vi "main_004.vi"() -> ()   [LabVIEW 2017]
uses:
  ISEGNHQxxu/iseg NHQ VISA Control.ctl
  <vilib>/Analysis/1siggen.llb/Ramp Pattern by Samples.vi
  <vilib>/Utility/file.llb/Read From Spreadsheet File (DBL).vi
  <vilib>/Utility/file.llb/Write Delimited Spreadsheet (string).vi
  <vilib>/Utility/file.llb/Write Delimited Spreadsheet (DBL).vi
  <vilib>/Platform/browser.llb/Open URL in Default Browser (path).vi
  <vilib>/Analysis/NI_AALBase.lvlib
  Newport ESP301/Newport ESP301.lvlib
panel:
  in  "continous acq.":bool
  in  "snap":bool
  in  "dark":bool
  in  "savebin":bool
  in  "savepng":bool
  in  "count?":bool
  in  "dark?":bool
  in  "threshold":i32=100
  in  "t_exp":dbl=0.10000637173652649 caption="Exposure time [s]"
  in  "dark_load":bool
  in  "frames":i32=300
  in  "avg[t] acc[f]":bool
  in  "Value in":dbl=2.0 caption="binning"
  in  "stop":bool
  out "Slide":dbl(slide)=0.9966666666666667 scale=0.0..1.0
  in  "open base path":bool
  in  "Path":path=path "W:/fsPPM/data/2019/11/191112"
  in  "Tab Control":T1(tab)=enum."delayscan"
  out "Waveform Chart":dbl(graph)=8402498.700000005
  in  "array size":i32=50
  out "noise-o-meter":dbl=7.252741087138157 format="%.1g"
  out "Actual Voltage":dbl[unit]=-90.03 format="%.2f"
  in  "volt_set":bool
  in  "Nominal Voltage":sgl=90.0 min=0 max=1000 step=1 format="%.2f"
  out "delayscan_time/step":dbl format="%.2f"
  out "delayscan_steps":i32
  in  "esp_rel_delta_fs":dbl=0.015 caption="delta [fs]" min=0.0
  in  "delayscan_go":bool
  in  "waypoints":string[][](table)=[["-500", "50"], ["500", ""], ["", ""]]
  in  "delayscan_header":string="DelayScan01" caption="header"
  in  "iterations":i32=1
  out "XY Graph":cluster{"Array":dbl[], dbl[]}(graph)={"Array"=[-500.0, -450.0, -400.0, -350.0, -300.0, -250.0, -200.0, -150.0, -100.0, -50.0, 0.0, 50.0, 100.0, 150.0, 200.0, 250.0, 300.0, 350.0, 400.0, 450.0, 500.0], [74.7680418855, 74.77553669695, 0.0, 0.0, 0.0, 0.0, 0.0, 0.0, 0.0, 0.0, 0.0, 0.0, 0.0, 0.0, 0.0, 0.0, 0.0, 0.0, 0.0, 0.0, 0.0]}
  in  "delayscan_stop":bool
  in  "esp_abs_dest":dbl=74.87296924580001 caption="[mm]"
  out "t0 @":dbl=74.84299 format="%.6g"
  in  "esp_set_t0":bool
  in  "esp_abs_time":dbl=200.0 caption="[fs]"
  in  "esp_rel_delta":dbl=0.015 caption="delta [mm]" min=0.0
  in  "esp_abs_go":bool
  in  "esp_rel-":bool
  in  "esp_rel+":bool
  out "delay_pos":dbl=74.77555 caption="[mm]" format="%.6g"
  out "esp_pos_fs":dbl=-449.91125160329966 caption="[fs]" format="%.6g"
  in  "delayscan_pause":bool caption="pause"
  out "duration":dbl format="%<%H:%M:%S>t"
  out "Slide 2":dbl(slide)=0.999 scale=0.0..1.0
  in  "meas_stop_volt":bool
  in  "meas_start_volt":bool
  in  "head":string="PowerVoltScan1"
  in  "volt_start":dbl format="%0.2f"
  in  "volt_end":dbl=1.0 format="%0.2f"
  in  "volt_samples":i32=128
  in  "iterations 2":i32
  in  "move2com":bool
  in  "meas_start_XY":bool
  in  "showcom":bool
  in  "VISA ISEG":refnum<visa-resource-name>="COM3"
  in  "Channel (A)":enum16{"A", "B"}(ring)=enum."B"
  out "error out":errorcluster
  in  "volt_timeout":u32=6000
  in  "volt_threshold":sgl=2.0 max=4000 format="%.2f"
  in  "esp_axis":i32=1 caption="ESP Axis" min=1 max=3
  in  "esp_visa":refnum<visa-resource-name>="COM2" caption="ESP VISA"
  out "esp301":errorcluster
  in  "Serial Link (RS232)":enum16{"RS232", "USB"}(ring)
  out "captured":dbl[][](graph)
  out "live":dbl[][](graph)
  in  "close":bool
  # "camera"
  # "voltage supply"
  # "Move absolute"
  # "Move relative"
  # "Axis1"
  # "Axis2"
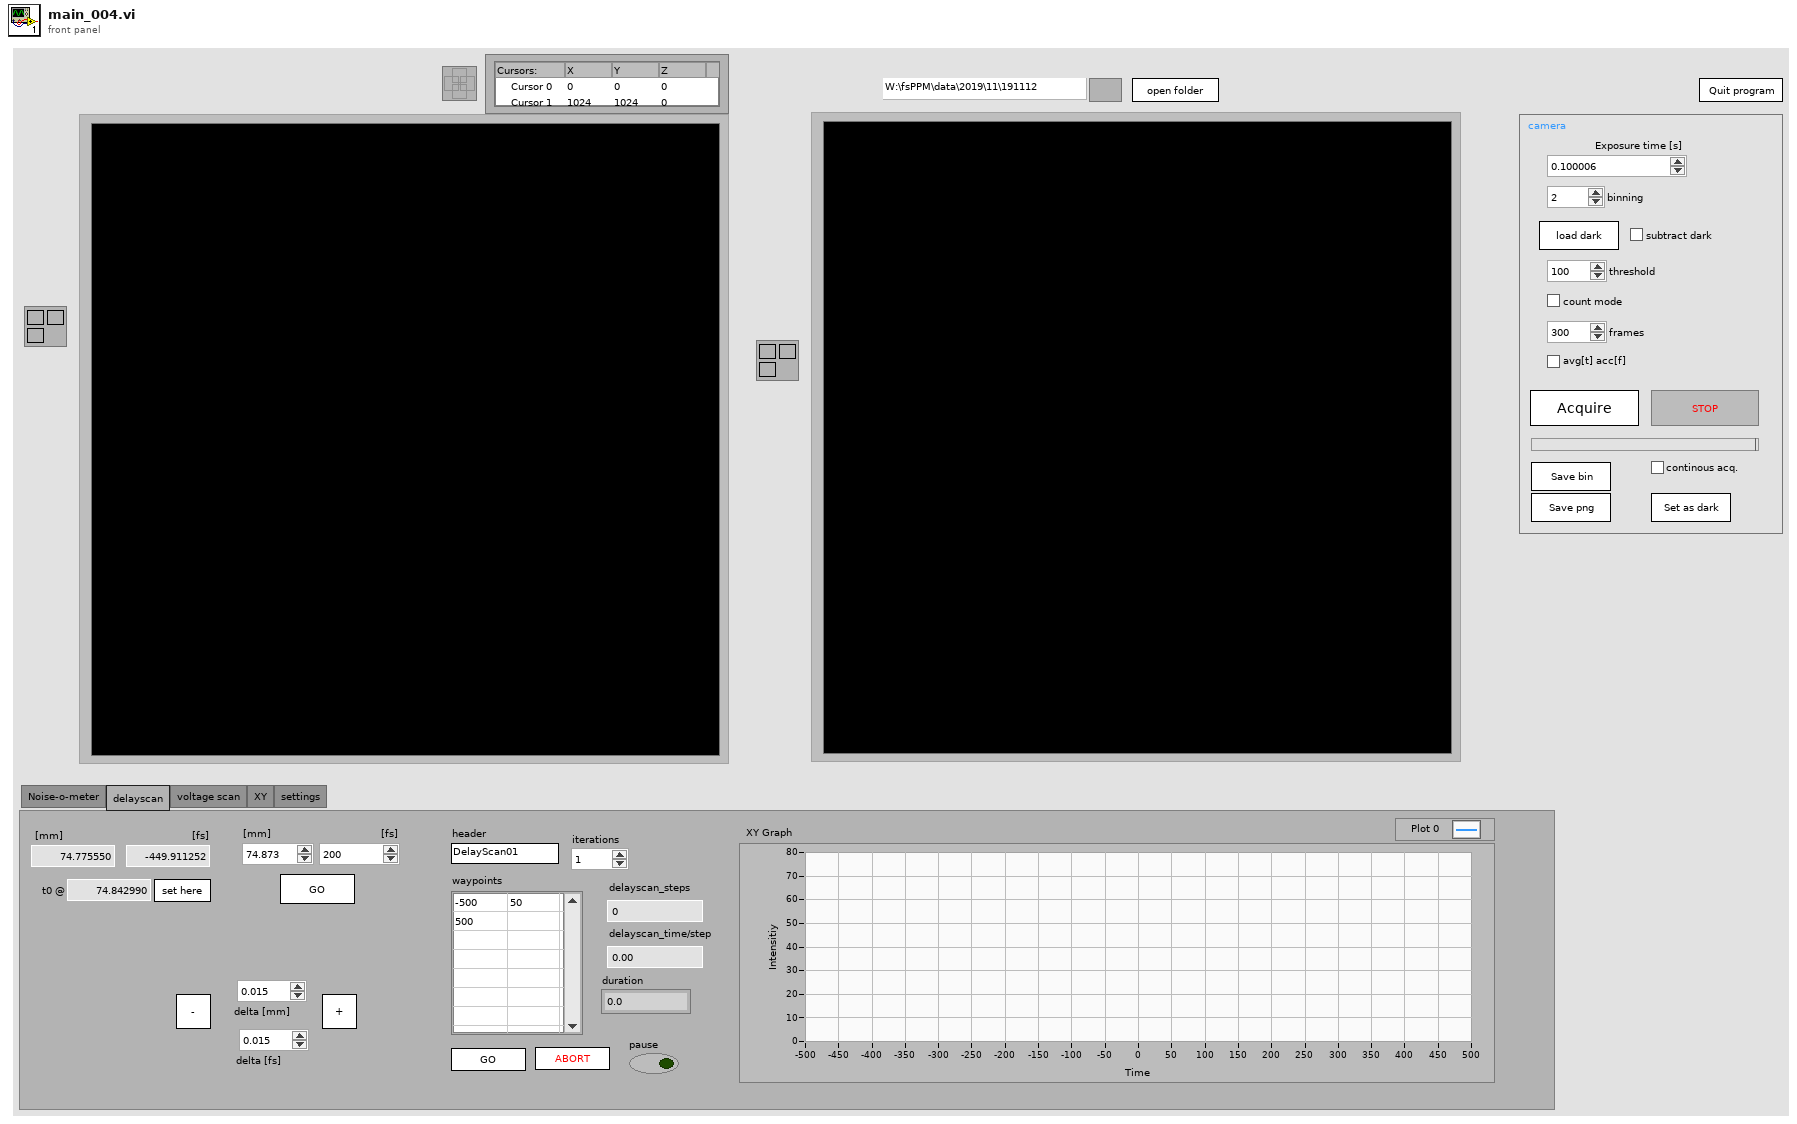
[diagram p1: front panel]
types:
  T1 = enum32{"Noise-o-meter", "delayscan", "voltage scan", "XY", "settings"}
  T2 = typedef "Image Type" = u32
  T3 = typedef "IMAQ Image.ctl" = refnum<image>
  T4 = cluster{"height":u32, "width":u32, "datatype":u32}
  T5 = cluster{"Axis1 moving":bool, "Axis2 moving":bool, "Axis3 moving":bool, "Axis4 moving":bool, "Motor Power of at least one axis":bool, "Reserved":bool, "Reserved":bool, "Reserved":bool, "Axis5 moving 2":bool, "Axis6 moving 2":bool, "Reserved":bool, "Reserved":bool, "Motor Power of at least one axis":bool, "Reserved":bool, "Reserved":bool, "Reserved":bool}
  T6 = typedef "iseg NHQ VISA Control.ctl" = cluster{"VISA Resource Name":refnum<visa-resource-name>, "FP Notation":bool, "Maximum Voltage":u32, "Maximum Current":u32}
  T7 = typedef "LVCursorListTypeDef.ctl" = cluster{"Name":string, "Color":u32, "Style":u8, "Point Style":u8, "Name Visible":bool, "Allow Drag":bool, "Cursor Mode":u32, "Plot":i32, "Index":i32, "Position":cluster{"X":dbl, "Y":dbl}, "X Scale":u32, "Y Scale":u32, "Watch Plots":i32[], "Watch All Plots":bool, "Plot Area":i32, "Label Offset":cluster{"X":dbl, "Y":dbl}}[]
  T8 = cluster{"Name":string, "Color":u32, "Style":u8, "Point Style":u8, "Name Visible":bool, "Allow Drag":bool, "Cursor Mode":u32, "Plot":i32, "Index":i32, "Position":cluster{"X":dbl, "Y":dbl}, "X Scale":u32, "Y Scale":u32, "Watch Plots":i32[], "Watch All Plots":bool, "Plot Area":i32, "Label Offset":cluster{"X":dbl, "Y":dbl}}
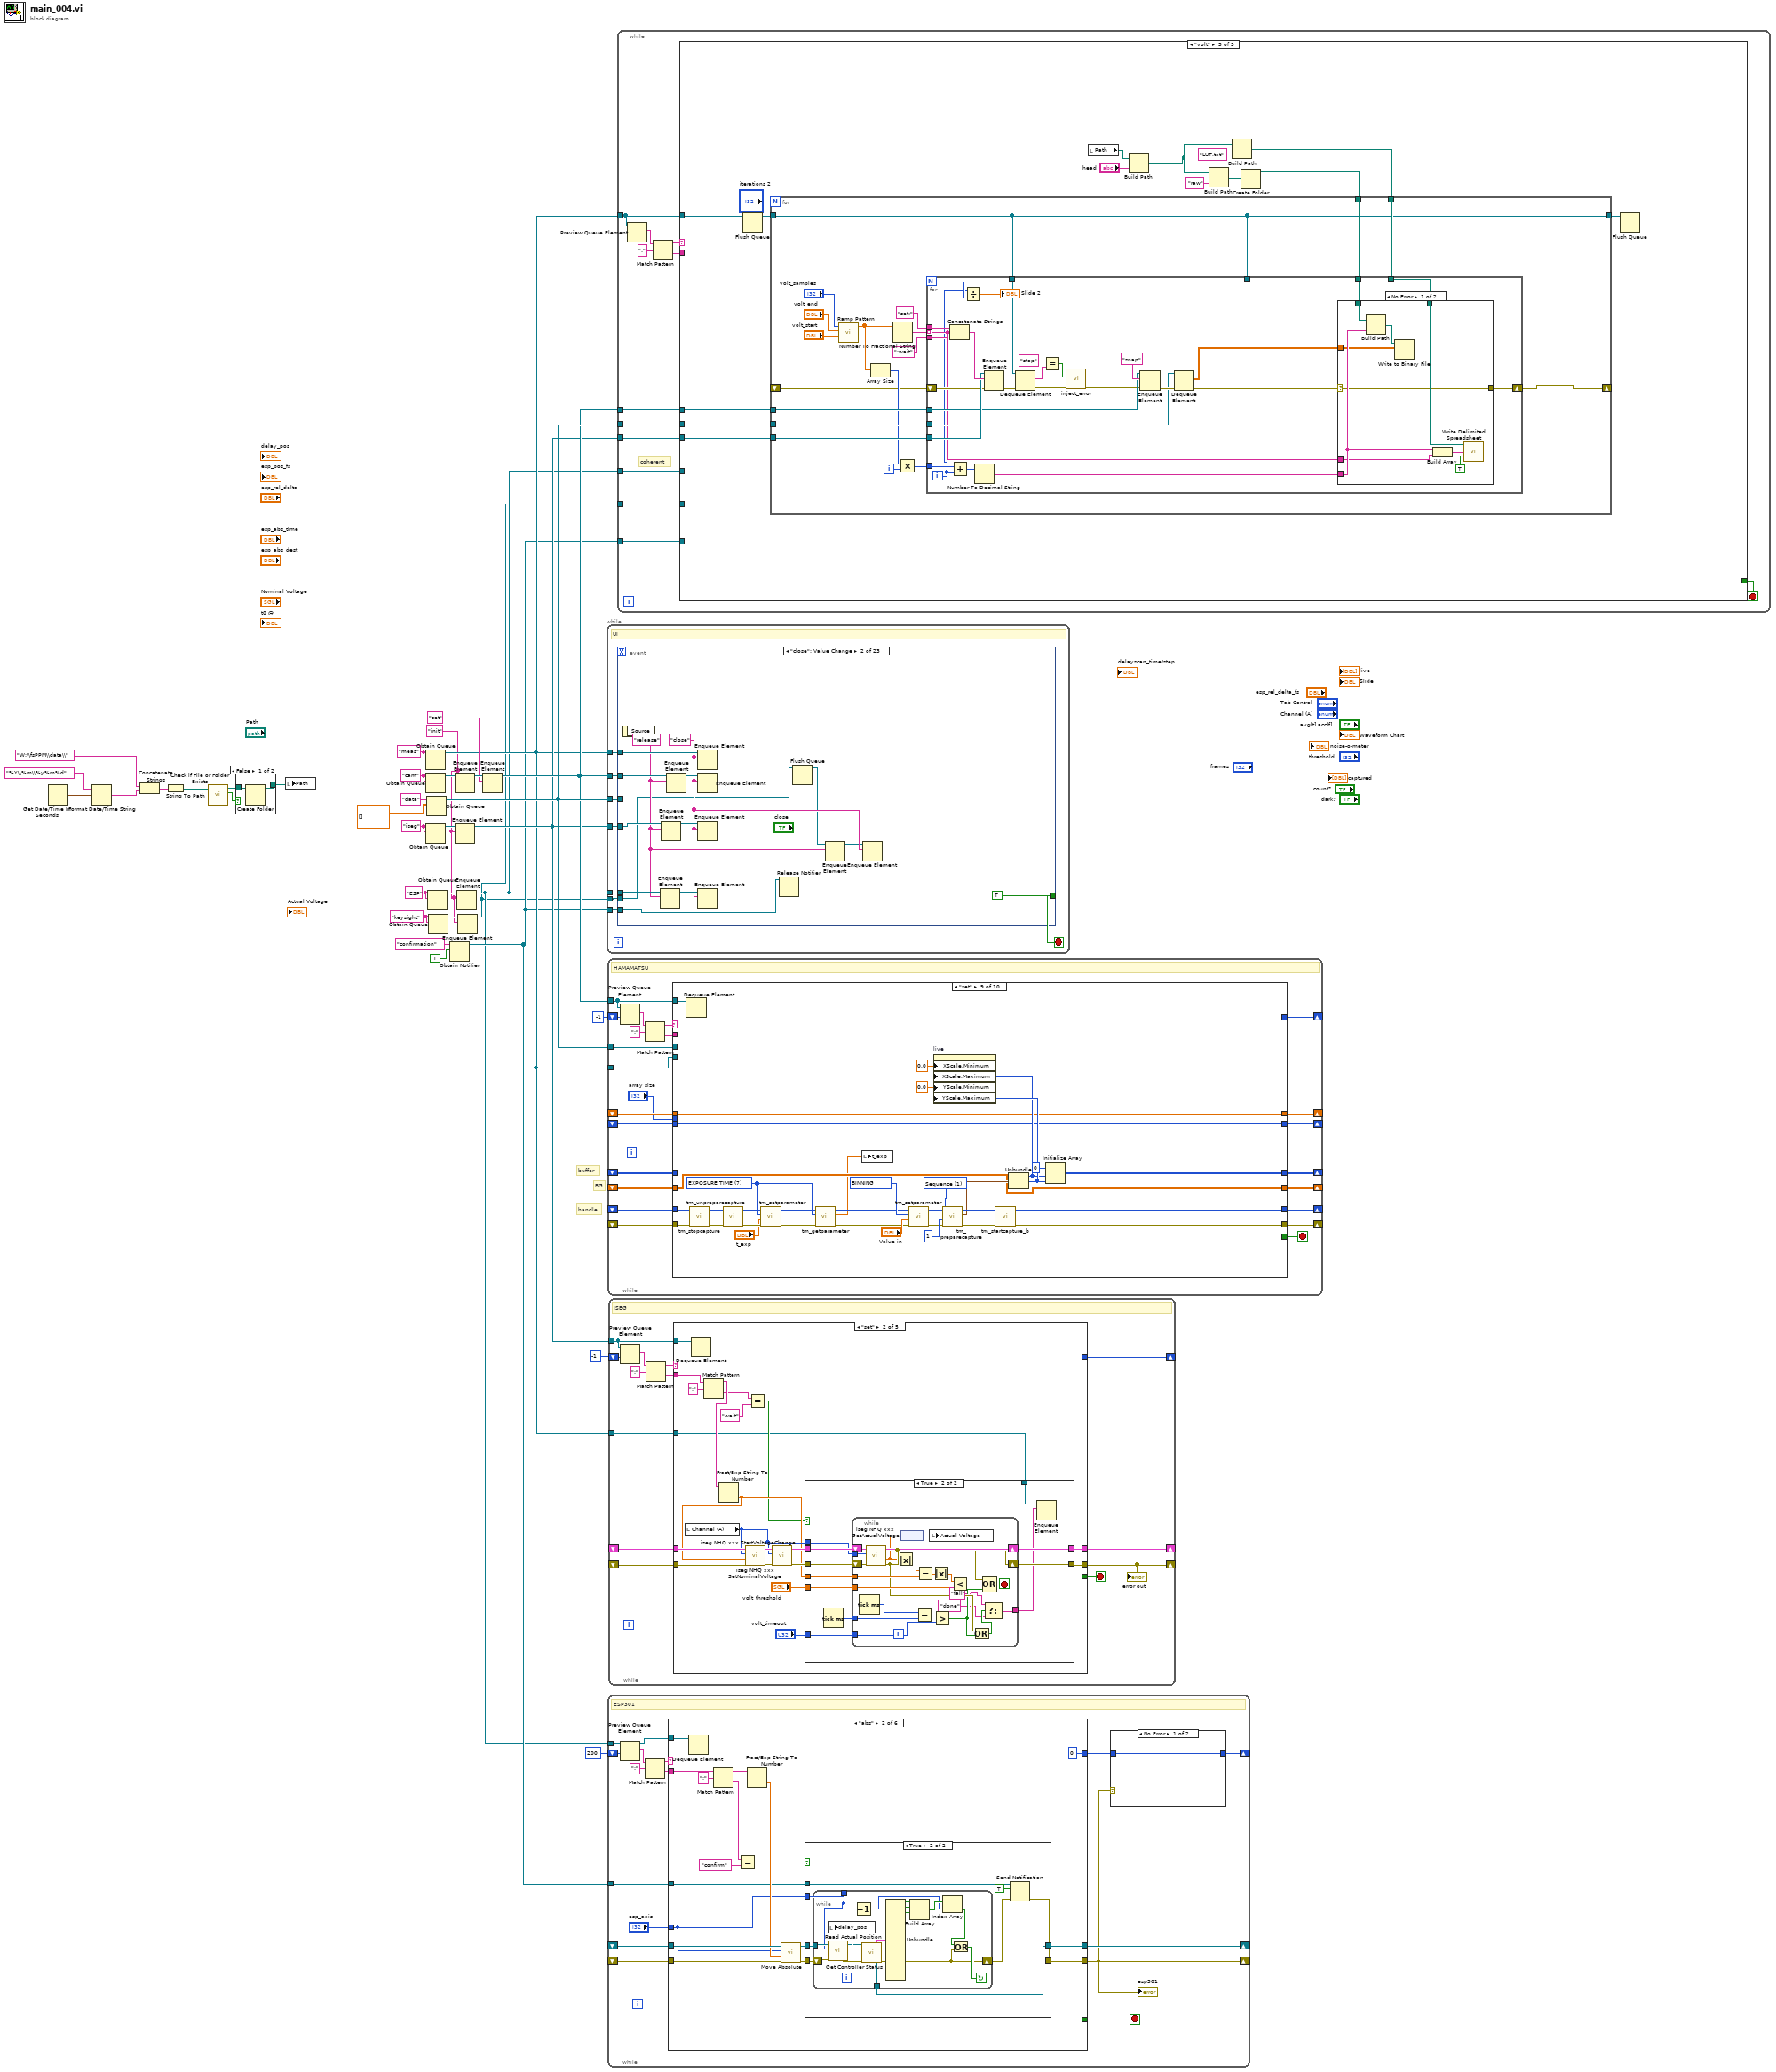
[diagram p0: block diagram]
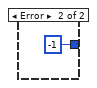
[diagram p3: hidden frame]
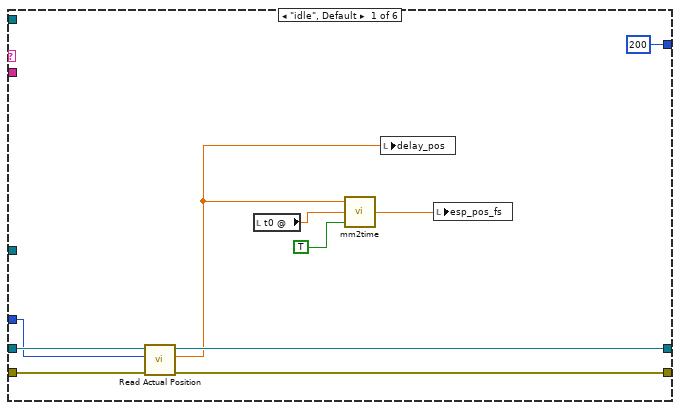
[diagram p4: hidden frame]
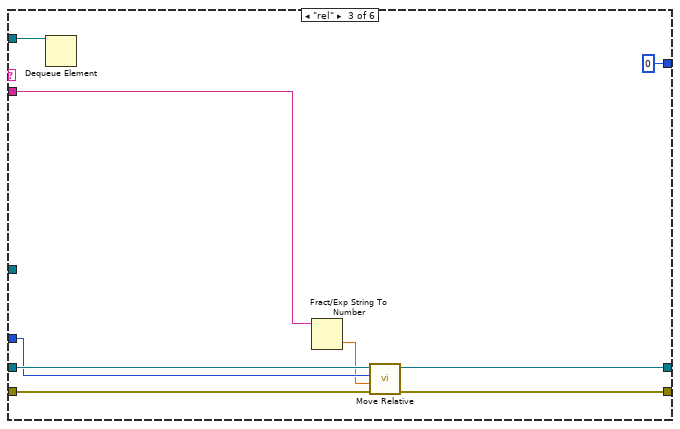
[diagram p6: hidden frame]
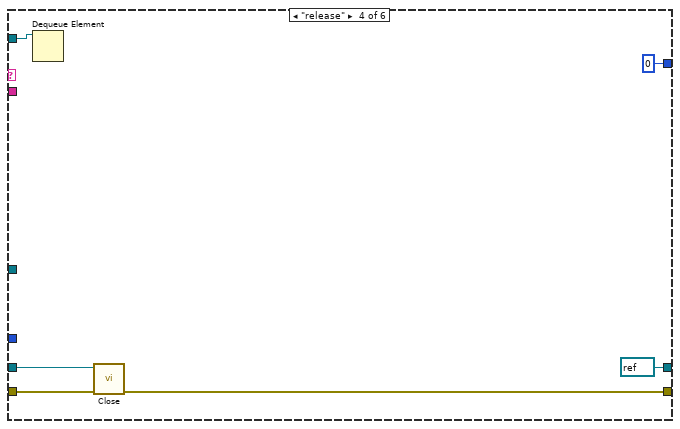
[diagram p7: hidden frame]
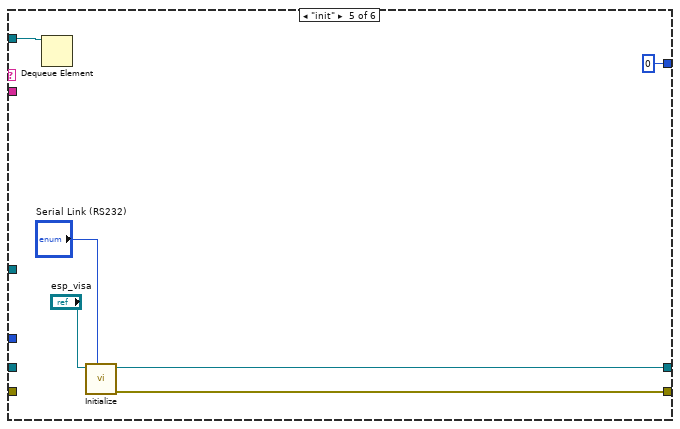
[diagram p8: hidden frame]
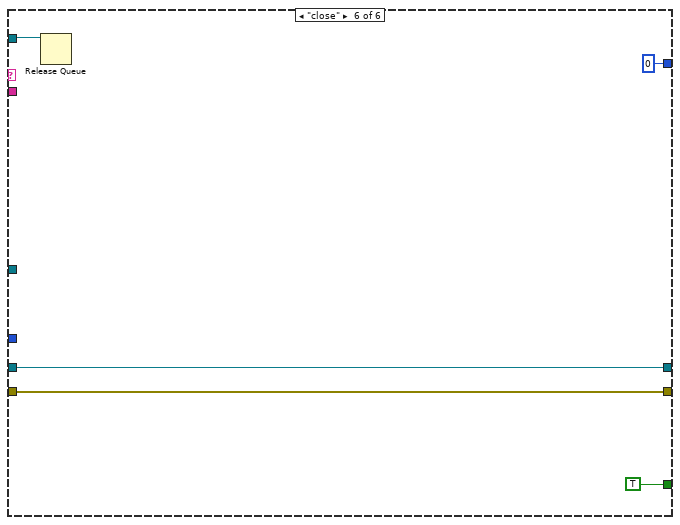
[diagram p9: hidden frame]
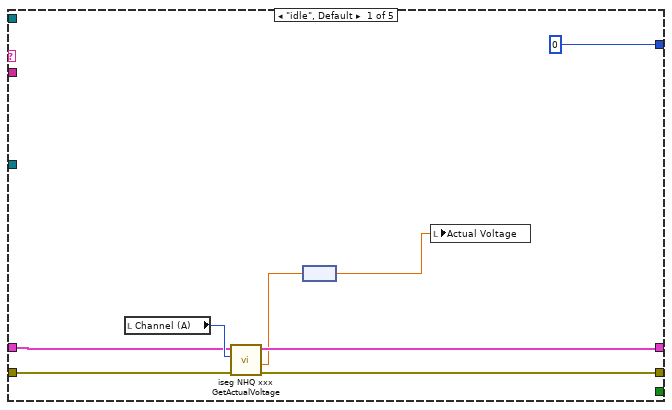
[diagram p10: hidden frame]
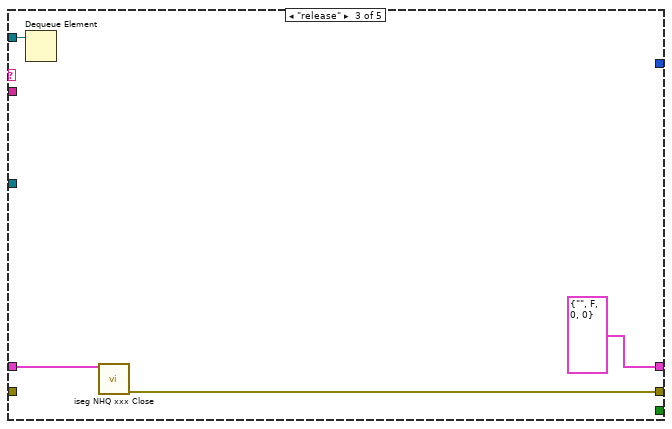
[diagram p12: hidden frame]
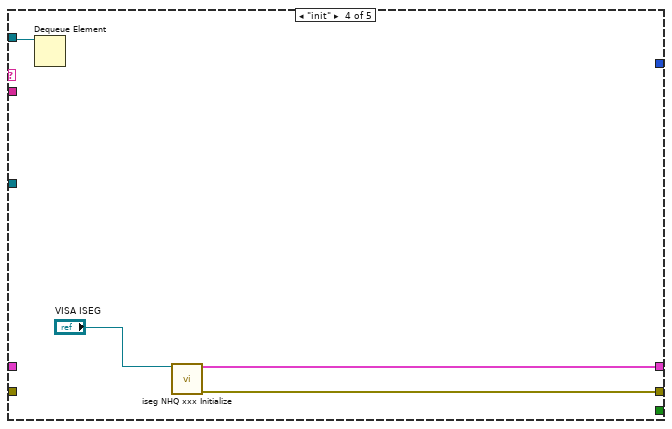
[diagram p13: hidden frame]
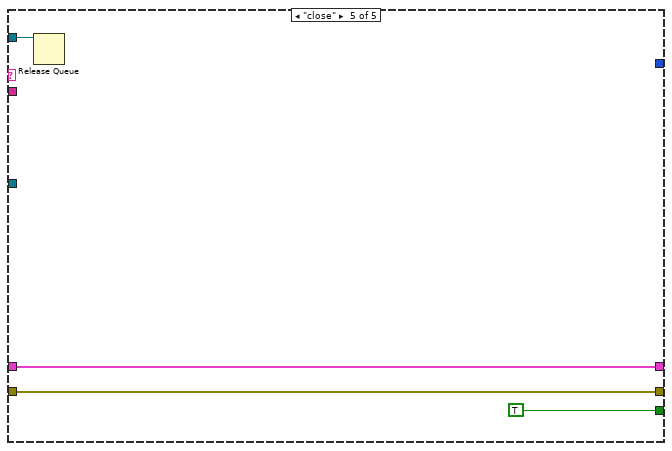
[diagram p14: hidden frame]
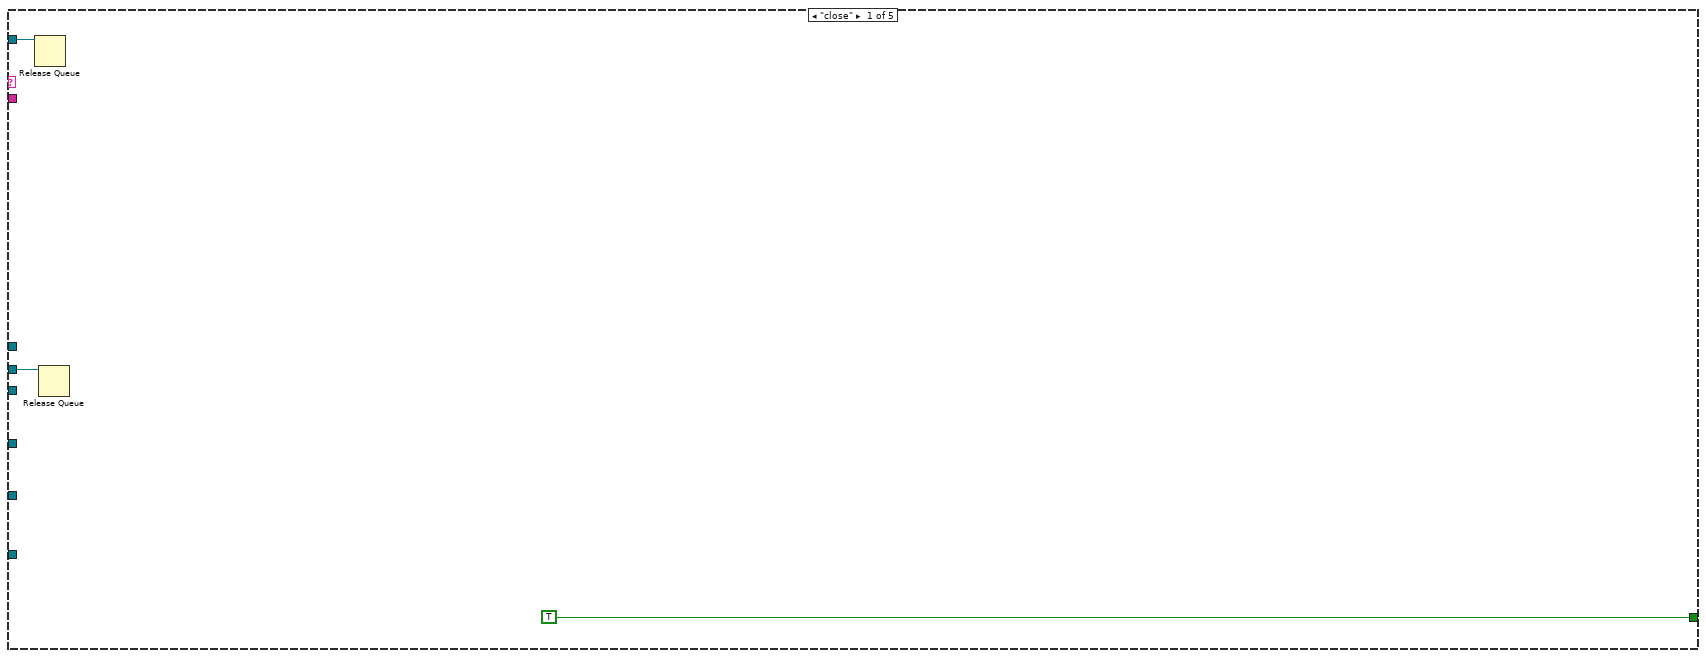
[diagram p15: hidden frame]
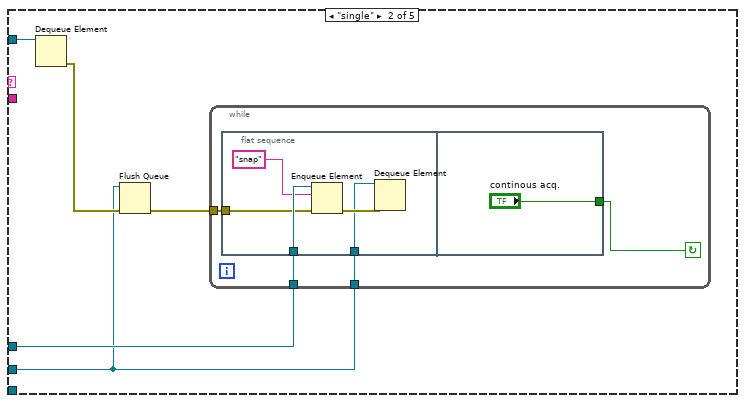
[diagram p16: hidden frame]
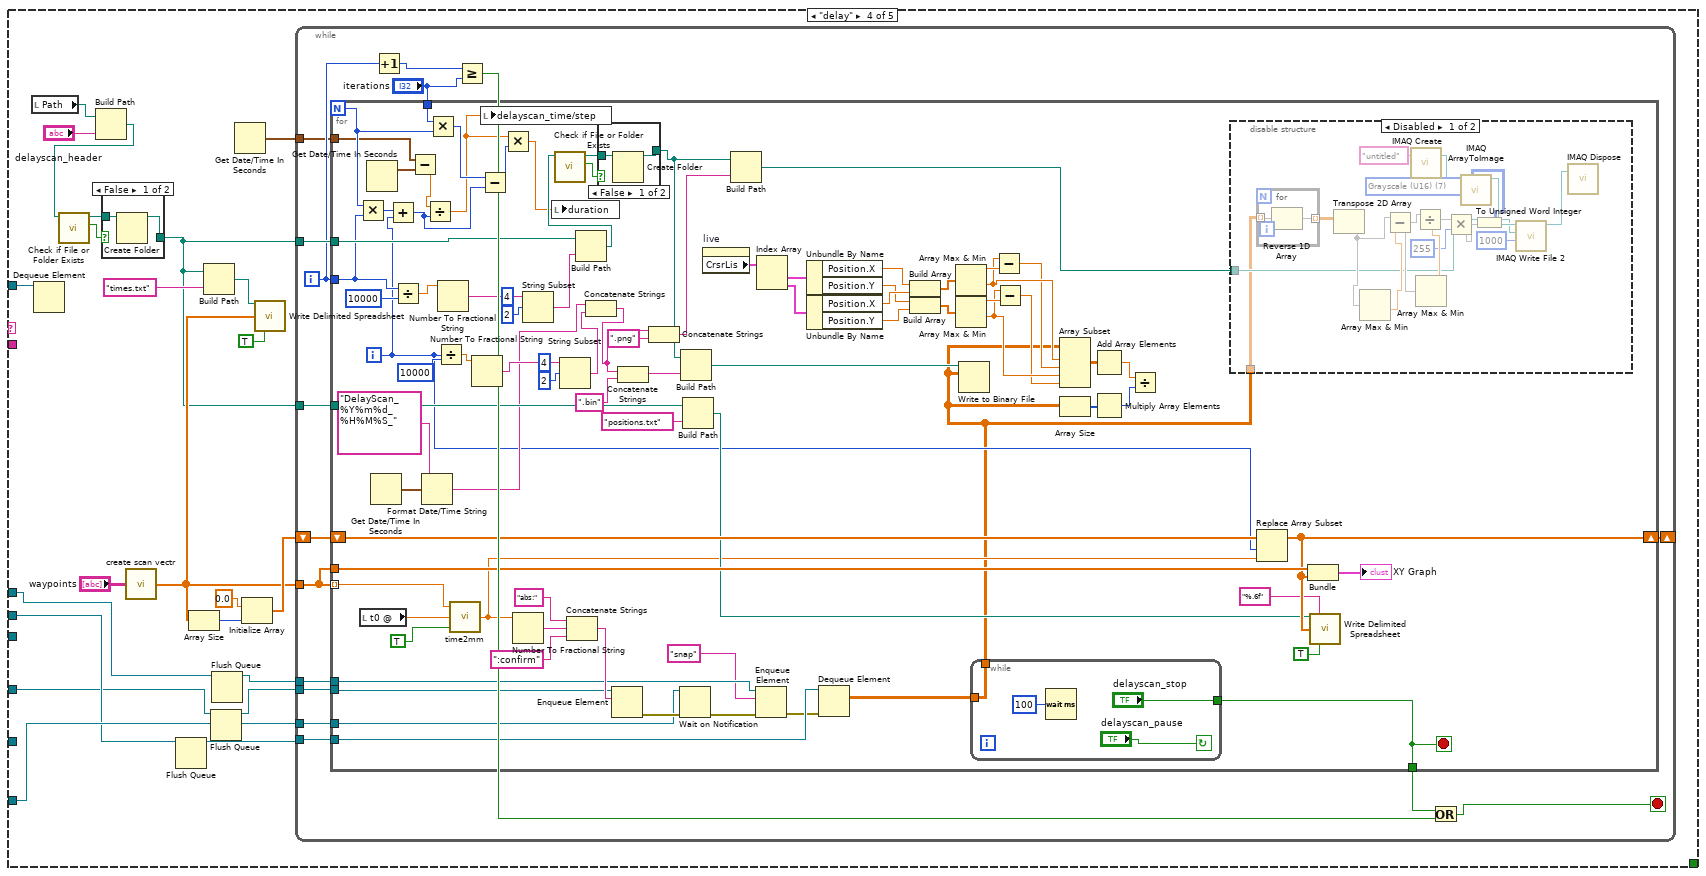
[diagram p18: hidden frame]
diagram:
  w3 = "keysight" ("name (unnamed)")
  w17 = "ESP" ("name (unnamed)")
  w25 = "iseg" ("name (unnamed)")
  w2 = "init" ("element")
  w32 = "meas" ("name (unnamed)")
  w33 = "cam" ("name (unnamed)")
  # "BG"
  # "handle"
  # "buffer"
  n1 = Get Date/Time In Seconds() -> (seconds since 1Jan1904=w14:timestamp)
  n2 = Format Date/Time String(time format string (%c)="%Y\\%m\\%y%m%d", seconds (now)=w14) -> (date/time string=w12:string)  [unwired: 1 in]
  n3 = Concatenate Strings("W:\\fsPPM\\data\\" ("string"), w12) -> (w10:string)
  n4 = String To Path(string=w10) -> (path=w7:path)
  n5 = call <vilib>:"Check if File or Folder Exists.vi"("path"=w7) -> ("file or folder exists?"=w9:bool, "dup path"=w8:path)  [unwired: 8 in, 1 out]
  n6 = case shown="False" w9 {
    tunnel: [w37 w38] -> w6
    tunnel: w8 -> [w36 w38]
    frame False {
      n7 = Create Folder(path (use dialog)=w36) -> (created path=w37:path)  [unwired: 2 in, 2 out]
    }
    frame True {
    }
  }
  n8 = local write "Path"(w6) -> ()
  n9 = Obtain Queue(name (unnamed)=w32, element data type=w32) -> (queue out=w21:refnum<queue>)  [unwired: 3 in, 2 out]
  n10 = Obtain Queue(name (unnamed)=w33, element data type=w33) -> (queue out=w35:refnum<queue>)  [unwired: 3 in, 2 out]
  n11 = Obtain Queue(name (unnamed)=w25, element data type=w25) -> (queue out=w24:refnum<queue>)  [unwired: 3 in, 2 out]
  n12 = Obtain Queue(name (unnamed)="data", element data type=dbl[][] []) -> (queue out=w28:refnum<queue>)  [unwired: 3 in, 2 out]
  n13 = Obtain Queue(name (unnamed)=w17, element data type=w17) -> (queue out=w16:refnum<queue>)  [unwired: 3 in, 2 out]
  n14 = Obtain Queue(name (unnamed)=w3, element data type=w3) -> (queue out=w4:refnum<queue>)  [unwired: 3 in, 2 out]
  n15 = Obtain Notifier(name (unnamed)="confirmation", notification data type=TRUE) -> (notifier out=w18:refnum<notifier>)  [unwired: 2 in, 2 out]
  n16 = Enqueue Element(queue=w35, element=w2) -> (queue out=w31:refnum<queue>)  [unwired: 2 in, 2 out]
  n17 = Enqueue Element(queue=w24, element=w2) -> (queue out=w22:refnum<queue>)  [unwired: 2 in, 2 out]
  n18 = Enqueue Element(queue=w16, element=w2) -> (queue out=w15:refnum<queue>)  [unwired: 2 in, 2 out]
  n19 = Enqueue Element(queue=w4, element=w2) -> (queue out=w1:refnum<queue>)  [unwired: 2 in, 2 out]
  n20 = Enqueue Element(queue=w31, element="set") -> (queue out=w27:refnum<queue>)  [unwired: 2 in, 2 out]
  n21 = while {
    tunnel: w27 -> [w46]
    tunnel: w21 -> [w45]
    tunnel: w28 -> [w44]
    tunnel: w22 -> [w42]
    tunnel: w18 -> [w41]
    tunnel: w15 -> [w40]
    tunnel: w1 -> [w39]
    stop <- w43 stop-if-true
    # "UI"
    n22 = event shown="[1] \"close\": Value Change" {
      selector: _ -> [_ _ _ _ _ _ _ _ _ _ _ _ _ _ _ _ _ _ _ _ _ _ _]
      dyn-events: _ -> [_ _ _ _ _ _ _ _ _ _ _ _ _ _ _ _ _ _ _ _ _ _ _]
      timeout: _ -> [_ _ _ _ _ _ _ _ _ _ _ _ _ _ _ _ _ _ _ _ _ _ _]
      tunnel: w46 -> [_ w59 _ _ _ _ _ _ _ _ _ w102 w104 _ _ _ _ _ _ w155 _ _ _]
      tunnel: w45 -> [_ w60 _ _ _ _ _ _ _ w96 _ _ _ w105 w108 w109 _ _ w149 _ w162 w164 _]
      tunnel: w44 -> [_ _ _ _ _ _ _ _ _ _ _ _ _ _ _ _ _ _ _ _ _ _ _]
      tunnel: [_ TRUE _ _ _ _ _ _ _ _ _ _ _ _ _ _ _ _ _ _ _ _ _] -> w43
      tunnel: w42 -> [_ w56 _ _ _ _ _ _ _ _ _ _ _ _ _ _ _ _ _ _ _ _ w169]
      tunnel: w41 -> [_ w52 _ _ _ _ _ _ _ _ _ _ _ _ _ _ _ _ _ _ _ _ _]
      tunnel: w40 -> [_ w54 w66 w71 _ _ _ _ _ _ _ _ _ _ _ _ _ _ _ _ _ _ _]
      tunnel: w39 -> [_ w47 _ _ _ _ _ _ _ _ _ _ _ _ _ _ _ _ _ _ _ _ _]
      event Timeout {
        n23 = event-data() -> ()  [unwired: 1 in, 1 out]
      }
      event "close": Value Change {
        w50 = "close" ("element")
        w51 = "release" ("element")
        n24 = event-data() -> ()  [unwired: 1 in, 1 out]
        n25 = Enqueue Element(queue=w54, element=w51) -> (queue out=w53:refnum<queue>)  [unwired: 2 in, 2 out]
        n26 = Enqueue Element(queue=w56, element=w51) -> (queue out=w55:refnum<queue>)  [unwired: 2 in, 2 out]
        n27 = Enqueue Element(queue=w59, element=w51) -> (queue out=w58:refnum<queue>)  [unwired: 2 in, 2 out]
        n28 = Enqueue Element(queue=w60, element=w50) -> ()  [unwired: 2 in, 3 out]
        n29 = Enqueue Element(queue=w58, element=w50) -> ()  [unwired: 2 in, 3 out]
        n30 = Enqueue Element(queue=w55, element=w50) -> ()  [unwired: 2 in, 3 out]
        n31 = Enqueue Element(queue=w53, element=w50) -> ()  [unwired: 2 in, 3 out]
        n32 = Release Notifier(notifier=w52) -> ()  [unwired: 2 in, 3 out]
        n33 = Flush Queue(queue=w47) -> (queue out=w48:refnum<queue>)  [unwired: 1 in, 2 out]
        n34 = Enqueue Element(queue=w48, element=w51) -> (queue out=w49:refnum<queue>)  [unwired: 2 in, 2 out]
        n35 = Enqueue Element(queue=w49, element=w50) -> ()  [unwired: 2 in, 3 out]
      }
      event "esp_abs_go": Value Change {
        n36 = event-data() -> ()  [unwired: 1 in, 1 out]
        n37 = local read "esp_abs_dest"() -> (w62:dbl)
        n38 = Number To Fractional String(number=w62) -> (F-format string=w63:string)  [unwired: 3 in]
        n39 = Concatenate Strings("abs:" ("string"), w63, ":confirm" ("string")) -> (w65:string)
        n40 = Enqueue Element(queue=w66, element=w65) -> ()  [unwired: 2 in, 3 out]
      }
      event "esp_rel+", "esp_rel-": Value Change {
        n41 = event-data() -> ()  [unwired: 1 in, 1 out]
        n42 = local read "esp_rel_delta"() -> (w69:dbl)
        n43 = Negate(x=w69) -> (-x=w70:dbl)
        n44 = Select(t=w70, s="esp_rel-", f=w69) -> (s? t:f=w68:dbl)
        n45 = Number To Fractional String(number=w68) -> (F-format string=w73:string)  [unwired: 3 in]
        n46 = Concatenate Strings("rel:" ("string"), w73) -> (w72:string)
        n47 = Enqueue Element(queue=w71, element=w72) -> ()  [unwired: 2 in, 3 out]
      }
      event "esp_rel_delta_fs": Value Change {
        n48 = event-data() -> ()  [unwired: 1 in, 1 out]
        n49 = local read "esp_rel_delta_fs"() -> (w75:dbl)
        n50 = call "time2mm.vi"("fs[1]/ps[0]"=TRUE, "time"=w75) -> ("position (mm)"=w76:dbl)  [unwired: 1 in]
        n51 = local write "esp_rel_delta"(w76) -> ()
      }
      event "esp_rel_delta": Value Change {
        n52 = event-data() -> ()  [unwired: 1 in, 1 out]
        n53 = local read "esp_rel_delta"() -> (w79:dbl)
        n54 = call "mm2time.vi"("fs?"=TRUE, "distance (mm)"=w79) -> ("time in fs/ps seconds"=w78:dbl)  [unwired: 1 in]
        n55 = local write "esp_rel_delta_fs"(w78) -> ()
      }
      event "waypoints", "iterations", "frames": Value Change {
        n56 = event-data() -> ()  [unwired: 1 in, 1 out]
        n57 = local read "waypoints"() -> (w89:string[][])
        n58 = local read "frames"() -> (w84:i32)
        n59 = local read "t_exp"() -> (w83:dbl)
        n60 = local read "iterations"() -> (w86:i32)
        n61 = Multiply(x=w84, y=w83) -> (x*y=w82:dbl)
        n62 = call "create scan vectr.vi"("Table Control"=w89) -> ("Array"=w88:dbl[])
        n63 = Array Size(array=w88) -> (size(s)=w87:i32)
        n64 = Multiply(x=w87, y=w86) -> (x*y=w85:i32)
        "delayscan_steps" <- w85
        n65 = Multiply(x=w82, y=w85) -> (x*y=→"duration":dbl)
        n66 = local write "delayscan_time/step"(w82) -> ()
      }
      event "esp_set_t0": Value Change {
        n67 = event-data() -> ()  [unwired: 1 in, 1 out]
        n68 = local read "delay_pos"() -> (w90:dbl)
        n69 = local write "t0 @"(w90) -> ()
      }
      event "esp_abs_time": Value Change {
        n70 = event-data() -> ()  [unwired: 1 in, 1 out]
        n71 = local read "esp_abs_time"() -> (w91:dbl)
        n72 = local read "t0 @"() -> (w92:dbl)
        n73 = call "time2mm.vi"("fs[1]/ps[0]"=TRUE, "Offset (mm)"=w92, "time"=w91) -> ("position (mm)"=w93:dbl)
        n74 = local write "esp_abs_dest"(w93) -> ()
      }
      event "delayscan_go": Value Change {
        n75 = event-data() -> ()  [unwired: 1 in, 1 out]
        n76 = Enqueue Element(queue=w96, element="delay") -> ()  [unwired: 2 in, 3 out]
      }
      event "esp_abs_dest": Value Change {
        n77 = event-data() -> ()  [unwired: 1 in, 1 out]
        n78 = local read "esp_abs_dest"() -> (w100:dbl)
        n79 = local read "t0 @"() -> (w99:dbl)
        n80 = call "mm2time.vi"("fs?"=TRUE, "Offset (mm)"=w99, "distance (mm)"=w100) -> ("time in fs/ps seconds"=w97:dbl)
        n81 = local write "esp_abs_time"(w97) -> ()
      }
      event "dark": Value Change {
        n82 = event-data() -> ()  [unwired: 1 in, 1 out]
        n83 = Enqueue Element(queue=w102, element="dark") -> ()  [unwired: 2 in, 3 out]
      }
      event "t_exp": Value Change {
        n84 = event-data() -> ()  [unwired: 1 in, 1 out]
        n85 = Enqueue Element(queue=w104, element="set") -> ()  [unwired: 2 in, 3 out]
      }
      event "snap": Value Change {
        n86 = event-data() -> ()  [unwired: 1 in, 1 out]
        n87 = Enqueue Element(queue=w105, element="single") -> ()  [unwired: 2 in, 3 out]
      }
      event "meas_start_volt": Value Change {
        n88 = event-data() -> ()  [unwired: 1 in, 1 out]
        n89 = Enqueue Element(queue=w108, element="volt") -> ()  [unwired: 2 in, 3 out]
      }
      event "meas_stop_volt": Value Change {
        n90 = event-data() -> ()  [unwired: 1 in, 1 out]
        n91 = Enqueue Element(queue=w109, element="stop") -> ()  [unwired: 2 in, 3 out]
      }
      event "open base path": Value Change {
        n92 = event-data() -> ()  [unwired: 1 in, 1 out]
        n93 = local read "Path"() -> (w111:path)
        n94 = call-poly <vilib>:"Open URL in Default Browser.vi"("path"=w111) -> ()  [unwired: 5 in, 2 out]
      }
      event "savebin", "savepng": Value Change {
        n95 = event-data() -> ()  [unwired: 1 in, 1 out]
        n96 = Get Date/Time In Seconds() -> (seconds since 1Jan1904=w117:timestamp)
        n97 = local read "Path"() -> (w113:path)
        n98 = Format Date/Time String(time format string (%c)="MCPIMG_%Y%m%d_%H%M%S", seconds (now)=w117) -> (date/time string=w112:string)  [unwired: 1 in]
        n99 = local read "captured"() -> (w114:dbl[][])
        n100 = case shown="False" "savebin" {
          tunnel: w114 -> [w132 w148]
          tunnel: w113 -> [w129 w142]
          tunnel: w112 -> [w127 w143]
          frame False {
            w137 = T2 7 items=["Grayscale (U8)", "Grayscale (I16)", "Grayscale (SGL)", "Complex (CSG)", "RGB (U32)", "HSL (U32)", "RGB (U64)", "Grayscale (U16)"] ("Image Type")
            n101 = for {
              tunnel: w132 -> [w140] mode=indexing
              tunnel: [w139] -> w131 mode=indexing
              n102 = Reverse 1D Array(array=w140) -> (reversed array=w139:dbl[])
            }
            n103 = Concatenate Strings(w127, ".png" ("string")) -> (w128:string)
            n104 = Transpose 2D Array(2D array=w131) -> (transposed array=w120:dbl[][])
            n105 = Array Max & Min(array=w120) -> (min value=w119:dbl)  [unwired: 3 out]
            n106 = Build Path(base path=w129, name or relative path=w128) -> (appended path=w130:path)
            n107 = Subtract(x=w120, y=w119) -> (x-y=w118:dbl[][])
            n108 = call "IMAQ Create"("Image Name"="untitled", "Image Type"=w137) -> ("New Image"=w138:T3)  [unwired: 3 in, 1 out]
            n109 = Array Max & Min(array=w118) -> (max value=w125:dbl)  [unwired: 3 out]
            n110 = Divide(x=w118, y=w125) -> (x/y=w124:dbl[][])
            n111 = Multiply(x=w124, y=255) -> (x*y=w122:dbl[][])
            n112 = To Unsigned Word Integer(number=w122) -> (unsigned 16bit integer=w121:u16[][])
            n113 = call "IMAQ ArrayToImage"("Image Pixels (U16)"=w121, "Image"=w138) -> ("Image Out"=w136:T3)  [unwired: 8 in, 1 out]
            n114 = call-poly "IMAQ Write File 2"("Image Quality"=u32 1000, "File Path"=w130, "Image"=w136) -> ("Image Out (duplicate)"=w134:T3)  [unwired: 7 in, 1 out]
            n115 = call "IMAQ Dispose"("Image"=w134) -> ()  [unwired: 5 in, 1 out]
          }
          frame True {
            n116 = Concatenate Strings(w143, ".bin" ("string")) -> (w145:string)
            n117 = Build Path(base path=w142, name or relative path=w145) -> (appended path=w141:path)
            n118 = Write to Binary File(file (use dialog)=w141, data=w148) -> (refnum out=w147:refnum<file>, error out=w146:errorcluster)  [unwired: 4 in, 1 out]
            n119 = Close File(refnum=w147, error in=w146) -> ()  [unwired: 2 out]
          }
        }
      }
      event "meas_start_XY": Value Change {
        n120 = event-data() -> ()  [unwired: 1 in, 1 out]
        n121 = Enqueue Element(queue=w149, element="XY") -> ()  [unwired: 2 in, 3 out]
      }
      event "dark_load": Value Change {
        n122 = event-data() -> ()  [unwired: 1 in, 1 out]
        n123 = local read "Path"() -> (w154:path)
        n124 = call "File Dialog"("start path"=w154) -> ("selected path"=w152:path, "cancelled"=w151:bool)  [unwired: 11 in, 2 out]
        n125 = case shown="False" w151 {
          tunnel: w155 -> [w160 _]
          tunnel: "dark_load:" ("element") -> [w158 _]
          tunnel: w152 -> [w156 _]
          frame False {
            n126 = Path To String(path=w156) -> (string=w157:string)
            n127 = Concatenate Strings(w158, w157) -> (w159:string)
            n128 = Enqueue Element(queue=w160, element=w159) -> ()  [unwired: 2 in, 3 out]
          }
          frame True {
          }
        }
      }
      event "move2com": Value Change {
        n129 = event-data() -> ()  [unwired: 1 in, 1 out]
        n130 = Enqueue Element(queue=w162, element="mov2cursor") -> ()  [unwired: 2 in, 3 out]
      }
      event "showcom": Value Change {
        n131 = event-data() -> ()  [unwired: 1 in, 1 out]
        n132 = Enqueue Element(queue=w164, element="showcom") -> ()  [unwired: 2 in, 3 out]
      }
      event "volt_set": Value Change {
        n133 = event-data() -> ()  [unwired: 1 in, 6 out]
        n134 = local read "Nominal Voltage"() -> (w165:sgl)
        n135 = Number To Fractional String(number=w165) -> (F-format string=w166:string)  [unwired: 3 in]
        n136 = Concatenate Strings("set:" ("element"), w166) -> (w168:string)
        n137 = Enqueue Element(queue=w169, element=w168) -> ()  [unwired: 2 in, 3 out]
      }
    }
  }
  n138 = while {
    tunnel: w27 -> [w188]
    shift-right: [w186] -> _
    shift-left: _ -> [w185]
    shift-right: [w184] -> _
    shift-left: _ -> [w183]
    shift-right: [w182] -> _
    shift-left: _ -> [w181]
    shift-right: [w180] -> _
    shift-left: _ -> [w179]
    shift-right: [w177] -> _
    shift-left: -1 -> [w178]
    tunnel: w28 -> [w176]
    tunnel: w21 -> [w175]
    shift-right: [w174] -> _
    shift-left: _ -> [w173]
    shift-right: [w171] -> _
    shift-left: _ -> [w172]
    stop <- w187 stop-if-true
    # "HAMAMATSU"
    n139 = Preview Queue Element(queue=w188, timeout in ms (-1)=w178) -> (element=w192:string)  [unwired: 1 in, 3 out]
    n140 = Match Pattern(string=w192, regular expression=":") -> (before substring=w190:string, after substring=w189:string)  [unwired: 1 in, 2 out]
    n141 = case shown="\"set\"" w190 {
      tunnel: w189 -> [_ _ w292 _ _ w382 _ _ _ _]
      tunnel: w188 -> [_ w231 w293 w327 w376 w386 w398 w401 w427 w449]
      tunnel: [_ _ _ _ _ _ _ _ _ TRUE] -> w187
      tunnel: [w211 w233 w296 w332 w374 w383 w390 w406 w415 w444] -> w186
      tunnel: w185 -> [w213 w236 w298 w334 w374 w383 w394 _ w441 w444]
      tunnel: [w212 w228 w297 w331 w373 w384 u32 0 ("Handle out") w404 w416 w445] -> w184
      tunnel: w183 -> [w214 w234 w299 w335 w373 w384 w395 _ w439 w445]
      tunnel: [w210 w235 w291 w330 w375 w385 w396 w402 w428 w446] -> w182
      tunnel: w181 -> [w210 w235 w291 w330 w375 w385 w396 w402 _ w446]
      tunnel: [w209 w232 w300 w333 w372 w379 w397 w403 w419 w447] -> w180
      tunnel: w179 -> [w209 w232 w300 w333 _ _ w397 w403 w419 w447]
      tunnel: [0 _ _ _ _ _ _ _ _ _] -> w177
      tunnel: w176 -> [_ w227 w301 _ _ _ _ _ _ _]
      tunnel: w175 -> [_ _ _ w328 _ _ _ _ _ _]
      tunnel: [w195 w222 w295 w319 w371 w378 w388 w400 w421 w443] -> w174
      tunnel: w173 -> [w204 w225 w295 w322 w371 w378 w388 w400 w421 w443]
      tunnel: w172 -> [w199 w224 w294 w320 w370 w377 w387 w399 w420 w442]
      tunnel: [w198 w221 w294 w318 w370 w377 w387 w399 w420 w442] -> w171
      tunnel: "array size" -> [w197 w223 _ w321 _ _ _ _ _ _]
      frame "idle", Default {
        n142 = local read "threshold"() -> (w215:i32)
        n143 = call "tm_getnextframe_a.vi"("error in (no error)"=w213, "Buffer"=w210, "Handle in"=w214) -> ("error out"=w211:errorcluster, "Data"=w205:u16[][], "Handle out"=w212:u32)  [unwired: 6 in]
        n144 = local read "dark?"() -> (w216:bool)
        n145 = local read "count?"() -> (w206:bool)
        n146 = case shown="False" w216 {
          tunnel: [w217 w220] -> w207
          tunnel: w205 -> [w217 w219]
          tunnel: w209 -> [_ w218]
          frame False {
          }
          frame True {
            n147 = Subtract(x=w219, y=w218) -> (x-y=w220:dbl[][])
          }
        }
        n148 = call "filtr_b.vi"("count?"=w206, "threshold"=w215, "input array"=w207) -> ("output array"=w193:dbl[][])  [unwired: 8 in]
        n149 = Add Array Elements(numeric array=w193) -> (sum=w194:dbl)
        n150 = call "ringbuffer.vi"("new val"=w194, "index in"=w199, "array size"=w197, "array in"=w204) -> ("index out"=w198:i32, "array out"=w195:dbl[])  [unwired: 6 in]
        n151 = local write "live"(w193) -> ()
        n152 = local write "Waveform Chart"(w194) -> ()
        n153 = call <vilib>:"Std Deviation and Variance.vi"("X"=w195) -> ("mean"=w200:dbl, "standard deviation"=w203:dbl)  [unwired: 1 in, 1 out]
        n154 = Divide(x=w203, y=w200) -> (x/y=w202:dbl)
        n155 = Multiply(x=w202, y=100.0) -> (x*y=w196:dbl)
        n156 = local write "noise-o-meter"(w196) -> ()
      }
      frame "snap" {
        n157 = Dequeue Element(queue=w231) -> ()  [unwired: 2 in, 4 out]
        n158 = local read "avg[t] acc[f]"() -> (w230:bool)
        n159 = local read "threshold"() -> (w238:i32)
        n160 = local read "frames"() -> (w237:i32)
        n161 = local read "count?"() -> (w229:bool)
        n162 = local read "dark?"() -> (w239:bool)
        n163 = for {
          N: w237 -> [w257]
          tunnel: w239 -> [w271]
          tunnel: w235 -> [w269]
          tunnel: w234 -> [w270]
          tunnel: w238 -> [w263]
          tunnel: [w267] -> w228
          shift-right: [w266] -> w233
          shift-left: w236 -> [w268]
          tunnel: w232 -> [w262]
          shift-right: [w240] -> w226
          shift-left: w235 -> [w260]
          tunnel: w230 -> [w261]
          tunnel: w229 -> [w259]
          shift-right: [w250] -> w222
          shift-left: w225 -> [w251]
          tunnel: w223 -> [w248]
          shift-right: [w247] -> w221
          shift-left: w224 -> [w249]
          shift-right: [w243] -> _
          shift-left: _ -> [w244]
          i -> [w258]
          stop <- "stop" stop-if-true
          n164 = call "tm_getnextframe_a.vi"("error in (no error)"=w268, "Buffer"=w269, "Handle in"=w270) -> ("error out"=w266:errorcluster, "Data"=w265:u16[][], "Handle out"=w267:u32)  [unwired: 6 in]
          n165 = Divide(x=w258, y=w257) -> (x/y=w256:dbl)
          n166 = case shown="True" w271 {
            tunnel: [w282 w285] -> w264
            tunnel: w265 -> [w282 w284]
            tunnel: w262 -> [_ w283]
            frame False {
            }
            frame True {
              n167 = Subtract(x=w284, y=w283) -> (x-y=w285:dbl[][])
            }
          }
          n168 = local write "Slide"(w256) -> ()
          n169 = Tick Count (ms)() -> (millisecond timer value=w243:u32)
          n170 = call "filtr_b.vi"("count?"=w259, "threshold"=w263, "input array"=w264) -> ("output array"=w242:dbl[][])  [unwired: 8 in]
          n171 = Subtract(x=w243, y=w244) -> ()  [unwired: 1 out]
          n172 = Add Array Elements(numeric array=w242) -> (sum=w241:dbl)
          n173 = call "ringbuffer.vi"("new val"=w241, "index in"=w249, "array size"=w248, "array in"=w251) -> ("index out"=w247:i32, "array out"=w250:dbl[])  [unwired: 6 in]
          n174 = call <vilib>:"Std Deviation and Variance.vi"("X"=w250) -> ("mean"=w252:dbl, "standard deviation"=w254:dbl)  [unwired: 1 in, 1 out]
          n175 = local write "live"(w242) -> ()
          n176 = local write "Waveform Chart"(w241) -> ()
          n177 = Divide(x=w254, y=w252) -> (x/y=w246:dbl)
          n178 = case shown="True" w261 {
            tunnel: w260 -> [w274 w281]
            tunnel: w242 -> [w273 w279]
            tunnel: [w272 w275] -> w240
            tunnel: w258 -> [_ w276]
            frame False {
              n179 = Add(x=w274, y=w273) -> (x+y=w272:dbl[][])
            }
            frame True {
              n180 = Multiply(x=w281, y=w276) -> (x*y=w280:dbl[][])
              n181 = Increment(x=w276) -> (x+1=w277:i32)
              n182 = Add(x=w280, y=w279) -> (x+y=w278:dbl[][])
              n183 = Divide(x=w278, y=w277) -> (x/y=w275:dbl[][])
            }
          }
          n184 = Multiply(x=w246, y=100.0) -> (x*y=w245:dbl)
          n185 = local write "noise-o-meter"(w245) -> ()
          n186 = local write "captured"(w240) -> ()
        }
        n187 = local write "captured"(w226) -> ()
        n188 = Enqueue Element(queue=w227, element=w226) -> ()  [unwired: 2 in, 3 out]
      }
      frame "single" {
        n189 = Dequeue Element(queue=w293) -> ()  [unwired: 2 in, 4 out]
        n190 = Decimal String To Number(string=w292) -> (number=w287:i32)  [unwired: 2 in, 1 out]
        n191 = To Unsigned Quad Integer(1:w291) -> (0:w290:u64[][])
        n192 = for {
          N: w287 -> [_]
          tunnel: w291 -> [w313]
          tunnel: w299 -> [w312]
          tunnel: w298 -> [w311]
          tunnel: [w310] -> w297
          tunnel: [w309] -> w296
          shift-right: [w306] -> w289
          shift-left: w290 -> [w308]
          n193 = call "tm_getnextframe_a.vi"("error in (no error)"=w311, "Buffer"=w313, "Handle in"=w312) -> ("error out"=w309:errorcluster, "Data"=w307:u16[][], "Handle out"=w310:u32)  [unwired: 6 in]
          n194 = Add(x=w307, y=w308) -> (x+y=w306:u64[][])
        }
        n195 = local read "dark?"() -> (w302:bool)
        n196 = Divide(x=w289, y=w287) -> (x/y=w288:dbl[][])
        n197 = case shown="True" w302 {
          tunnel: [w314 w317] -> w305
          tunnel: w288 -> [w314 w316]
          tunnel: w300 -> [_ w315]
          frame False {
          }
          frame True {
            n198 = Subtract(x=w316, y=w315) -> (x-y=w317:dbl[][])
          }
        }
        n199 = local read "threshold"() -> (w303:i32)
        n200 = local read "count?"() -> (w304:bool)
        n201 = call "filtr_b.vi"("count?"=w304, "threshold"=w303, "input array"=w305) -> ("output array"=w286:dbl[][])  [unwired: 8 in]
        n202 = Enqueue Element(queue=w301, element=w286) -> ()  [unwired: 2 in, 3 out]
        n203 = local write "captured"(w286) -> ()
      }
      frame "snap_I" {
        n204 = Dequeue Element(queue=w327) -> ()  [unwired: 2 in, 4 out]
        n205 = local read "threshold"() -> (w338:i32)
        n206 = local read "frames"() -> (w337:i32)
        n207 = local read "count?"() -> (w336:bool)
        n208 = local read "dark?"() -> (w339:bool)
        n209 = for {
          N: w337 -> [w353]
          tunnel: w339 -> [w365]
          tunnel: w330 -> [w363]
          tunnel: w335 -> [w364]
          tunnel: w338 -> [w357]
          tunnel: [w361] -> w331
          shift-right: [w360] -> w332
          shift-left: w334 -> [w362]
          tunnel: w333 -> [w356]
          tunnel: w336 -> [w355]
          tunnel: [w351] -> w329 mode=indexing
          shift-right: [w343] -> w319
          shift-left: w322 -> [w344]
          tunnel: w321 -> [w342]
          shift-right: [w340] -> w318
          shift-left: w320 -> [w341]
          i -> [w354]
          n210 = call "tm_getnextframe_a.vi"("error in (no error)"=w362, "Buffer"=w363, "Handle in"=w364) -> ("error out"=w360:errorcluster, "Data"=w359:u16[][], "Handle out"=w361:u32)  [unwired: 6 in]
          n211 = call "ringbuffer.vi"("index in"=w341, "array size"=w342, "array in"=w344) -> ("index out"=w340:i32, "array out"=w343:dbl[])  [unwired: 7 in]
          n212 = Divide(x=w354, y=w353) -> (x/y=w352:dbl)
          n213 = case shown="True" w365 {
            tunnel: [w366 w369] -> w358
            tunnel: w359 -> [w366 w368]
            tunnel: w356 -> [_ w367]
            frame False {
            }
            frame True {
              n214 = Subtract(x=w368, y=w367) -> (x-y=w369:dbl[][])
            }
          }
          n215 = local write "Slide"(w352) -> ()
          n216 = call <vilib>:"Std Deviation and Variance.vi"("X"=w343) -> ("mean"=w345:dbl, "standard deviation"=w348:dbl)  [unwired: 1 in, 1 out]
          n217 = call "filtr_b.vi"("count?"=w355, "threshold"=w357, "input array"=w358) -> ("output array"=w350:dbl[][])  [unwired: 8 in]
          n218 = Divide(x=w348, y=w345) -> (x/y=w347:dbl)
          n219 = local write "live"(w350) -> ()
          n220 = Multiply(x=w347, y=100.0) -> (x*y=w349:dbl)
          n221 = local write "noise-o-meter"(w349) -> ()
          n222 = Add Array Elements(numeric array=w350) -> (sum=w351:dbl)
          n223 = local write "Waveform Chart"(w351) -> ()
        }
        n224 = call <vilib>:"Std Deviation and Variance.vi"("X"=w329) -> ("mean"=w326:dbl, "standard deviation"=w325:dbl)  [unwired: 1 in, 1 out]
        n225 = Format Into String(format string="%.6e;%.6e", w326, w325) -> (resulting string=w324:string)  [unwired: 2 in, 1 out]
        n226 = Enqueue Element(queue=w328, element=w324) -> ()  [unwired: 2 in, 3 out]
      }
      frame "dark" {
        n227 = Dequeue Element(queue=w376) -> ()  [unwired: 2 in, 4 out]
        n228 = local read "captured"() -> (w372:dbl[][])
      }
      frame "dark_load" {
        n229 = Dequeue Element(queue=w386) -> ()  [unwired: 2 in, 4 out]
        n230 = String To Path(string=w382) -> (path=w381:path)
        n231 = Read from Binary File(5:dbl[][] [] ("all rows"), 11:w381) -> (2:w379:dbl[][])  [unwired: 4 in, 3 out]
        n232 = call-poly <vilib>:"Read From Spreadsheet File.vi"("file path (dialog if empty)"=w381) -> ()  [unwired: 6 in, 5 out]
      }
      frame "release" {
        n233 = call "tm_stopcapture.vi"("error in (no error)"=w394, "Handle in"=w395) -> ("error out"=w392:errorcluster, "Handle out"=w393:u32)  [unwired: 8 in]
        n234 = Dequeue Element(queue=w398) -> ()  [unwired: 2 in, 4 out]
        n235 = call "tm_closecamera.vi"("error in (no error)"=w392, "Handle in"=w393) -> ("error out"=w391:errorcluster)  [unwired: 9 in]
        n236 = call "tm_deinitialize.vi"("error in (no error)"=w391) -> ("error out"=w390:errorcluster)  [unwired: 10 in]
      }
      frame "init" {
        n237 = Dequeue Element(queue=w401) -> ()  [unwired: 2 in, 4 out]
        n238 = call "tm_initialize.vi"() -> ("error out"=w407:errorcluster)  [unwired: 8 in, 3 out]
        n239 = call "tm_opencamera.vi"("error in (no error)"=w407, "Camera Index"=u32 0) -> ("error out"=w406:errorcluster, "Handle out"=w404:u32)  [unwired: 7 in, 1 out]
      }
      frame "set" {
        w433 = 1 items=["Snap", "Sequence"] ("Capture mode")
        w434 = u32 4215968 items=["BINNING"=4215968, "BITS PER CHANNEL"=2, "ACTIVE VIEW INDEX"=3, "CCD MODE"=4, "SENSOR MODE"=5, "READOUT MODE"=6, "EXPOSURE TIME"=7, "CONTRAST GAIN"=8, "CONTRAST OFFSET"=9, "LIGHT MODE"=10, "SENSITIVITY"=11, "WHITE BALANCE"=12, "PHOTON IMAGING MODE"=13, "HIGH DYNAMIC RANGE MODE"=14, "TRIGGER SOURCE"=15, "TRIGGER ACTIVE"=16, "TRIGGER MODE"=17, "TRIGGER POLARITY"=18, "TRIGGER GLOBAL EXPOSURE"=19, "FIRST TRIGGER BEHAVIOR"=20, "TRIGGER TIMES"=21, "OUTPUT TRIGGER POLARITY"=22, "OUTPUT TRIGGER DELAY"=23, "OUTPUT TRIGGER PERIOD"=24, "TEMPERATURE"=25, "TEMPERATURE TARGET"=26, "SENSOR COOLER FAN"=27, "MECHANICAL SHUTTER"=28, "BACK FOCUS POSITION"=29, "FRAMEBUNDLE MODE"=30, "FRAMEBUNDLE NUMBER"=31, "LINEBUNDLE HEIGHT"=32, "TRIGGER CONNECTOR"=33, "IMAGE PIXEL TYPE"=34, "OUTPUT TRIGGER KIND"=35, "READOUT DIRECTION"=36, "CHANNEL SYNC"=37] ("Parameter")
        w411 = u32 7 items=["BINNING"=4215968, "BITS PER CHANNEL"=2, "ACTIVE VIEW INDEX"=3, "CCD MODE"=4, "SENSOR MODE"=5, "READOUT MODE"=6, "EXPOSURE TIME"=7, "CONTRAST GAIN"=8, "CONTRAST OFFSET"=9, "LIGHT MODE"=10, "SENSITIVITY"=11, "WHITE BALANCE"=12, "PHOTON IMAGING MODE"=13, "HIGH DYNAMIC RANGE MODE"=14, "TRIGGER SOURCE"=15, "TRIGGER ACTIVE"=16, "TRIGGER MODE"=17, "TRIGGER POLARITY"=18, "TRIGGER GLOBAL EXPOSURE"=19, "FIRST TRIGGER BEHAVIOR"=20, "TRIGGER TIMES"=21, "OUTPUT TRIGGER POLARITY"=22, "OUTPUT TRIGGER DELAY"=23, "OUTPUT TRIGGER PERIOD"=24, "TEMPERATURE"=25, "TEMPERATURE TARGET"=26, "SENSOR COOLER FAN"=27, "MECHANICAL SHUTTER"=28, "BACK FOCUS POSITION"=29, "FRAMEBUNDLE MODE"=30, "FRAMEBUNDLE NUMBER"=31, "LINEBUNDLE HEIGHT"=32, "TRIGGER CONNECTOR"=33, "IMAGE PIXEL TYPE"=34, "OUTPUT TRIGGER KIND"=35, "READOUT DIRECTION"=36, "CHANNEL SYNC"=37] ("Parameter")
        n240 = Dequeue Element(queue=w427) -> ()  [unwired: 2 in, 4 out]
        n241 = call "tm_stopcapture.vi"("error in (no error)"=w441, "Handle in"=w439) -> ("error out"=w440:errorcluster, "Handle out"=w438:u32)  [unwired: 8 in]
        n242 = call "tm_unpreparecapture.vi"("error in (no error)"=w440, "Handle in"=w438) -> ("error out"=w437:errorcluster, "Handle out"=w436:u32)  [unwired: 8 in]
        n243 = call "tm_setparameter.vi"("error in (no error)"=w437, "Value in"="t_exp", "Parameter"=w411, "Handle in"=w436) -> ("error out"=w413:errorcluster, "Handle out"=w412:u32)  [unwired: 6 in]
        n244 = call "tm_getparameter.vi"("error in (no error)"=w413, "Parameter"=w411, "Handle in"=w412) -> ("error out"=w409:errorcluster, "Value out"=w408:dbl, "Handle out"=w410:u32)  [unwired: 6 in]
        n245 = local write "t_exp"(w408) -> ()
        n246 = call "tm_setparameter.vi"("error in (no error)"=w409, "Value in"="Value in", "Parameter"=w434, "Handle in"=w410) -> ("error out"=w417:errorcluster, "Handle out"=w418:u32)  [unwired: 6 in]
        n247 = call "tm_preparecapture.vi"("error in (no error)"=w417, "Frames"=1, "Capture mode"=w433, "Handle in"=w418) -> ("error out"=w430:errorcluster, "Buffer Info"=w429:T4, "Handle out"=w431:u32)  [unwired: 4 in, 1 out]
        n248 = call "tm_startcapture_b.vi"("error in (no error)"=w430, "Handle in"=w431) -> ("error out"=w415:errorcluster, "Handle out"=w416:u32)  [unwired: 8 in]
        n249 = Unbundle(w429) -> ("height"=w425:u32, "width"=w426:u32)  [unwired: 1 out]
        n250 = property on="live" class="IntGraph (strict)"("XScale.Minimum"=0.0 ("X Scale.Range:Minimum"), "XScale.Maximum"=w425, "YScale.Minimum"=0.0 ("Y Scale.Range:Minimum"), "YScale.Maximum"=w426) -> ()  [unwired: 2 in, 2 out]
        n251 = Initialize Array(u16 0 ("element"), w425, w426) -> (w428:u16[][])
      }
      frame "close" {
        n252 = Release Queue(queue=w449) -> ()  [unwired: 2 in, 3 out]
      }
    }
  }
  n253 = while {
    shift-right: [w452] -> _
    shift-left: _ -> [w460]
    shift-right: [w458] -> _
    shift-left: 200 -> [w459]
    shift-right: [w456] -> _
    shift-left: _ -> [w455]
    tunnel: w18 -> [w453]
    tunnel: w15 -> [w450]
    stop <- w461 stop-if-true
    # "ESP301"
    n254 = Preview Queue Element(queue=w450, timeout in ms (-1)=w459) -> (queue out=w457:refnum<queue>, element=w465:string)  [unwired: 1 in, 2 out]
    n255 = Match Pattern(string=w465, regular expression=":") -> (before substring=w463:string, after substring=w462:string)  [unwired: 1 in, 2 out]
    n256 = case shown="\"abs\"" w463 {
      tunnel: w462 -> [_ w490 w530 _ _ _]
      tunnel: [_ _ _ _ _ TRUE] -> w461
      tunnel: [w474 w485 w526 w533 w541 w546] -> w452
      tunnel: w460 -> [w477 w494 w528 w535 _ w546]
      tunnel: w457 -> [_ w481 w522 w532 w542 w544]
      tunnel: [w475 w478 w527 refnum<visa-resource-name> refnum ("VISA resource name out") w540 w545] -> w456
      tunnel: w455 -> [w476 w493 w529 w536 _ w545]
      tunnel: "esp_axis" -> [w473 w479 w525 _ _ _]
      tunnel: w453 -> [_ w483 _ _ _ _]
      tunnel: [200 0 0 0 0 0] -> w451
      frame "idle", Default {
        n257 = call "Read Actual Position.vi"("error in (no error)"=w477, "Axis (1)"=w473, "VISA resource name"=w476) -> ("error out"=w474:errorcluster, "Position (units)"=w468:dbl, "VISA resource name out"=w475:refnum<visa-resource-name>)  [unwired: 2 in]
        n258 = local read "t0 @"() -> (w471:dbl)
        n259 = call "mm2time.vi"("fs?"=TRUE, "Offset (mm)"=w471, "distance (mm)"=w468) -> ("time in fs/ps seconds"=w469:dbl)
        n260 = local write "delay_pos"(w468) -> ()
        n261 = local write "esp_pos_fs"(w469) -> ()
      }
      frame "abs" {
        n262 = Dequeue Element(queue=w481) -> ()  [unwired: 2 in, 4 out]
        n263 = Match Pattern(string=w490, regular expression=":") -> (before substring=w489:string, after substring=w488:string)  [unwired: 1 in, 2 out]
        n264 = Equal?(x=w488, y="confirm") -> (x = y?=w484:bool)
        n265 = Fract/Exp String To Number(string=w489) -> (number=w492:dbl)  [unwired: 3 in, 1 out]
        n266 = call "Move Absolute.vi"("error in (no error)"=w494, "Position (0 units)"=w492, "Axis (1)"=w479, "VISA resource name"=w493) -> ("error out"=w486:errorcluster, "VISA resource name out"=w480:refnum<visa-resource-name>)  [unwired: 2 in]
        n267 = case shown="True" w484 {
          tunnel: w486 -> [w496 w501]
          tunnel: [w496 w504] -> w485
          tunnel: w483 -> [_ w503]
          tunnel: w480 -> [w495 w499]
          tunnel: w479 -> [_ w498]
          tunnel: [w495 w497] -> w478
          frame False {
          }
          frame True {
            n268 = while {
              tunnel: w499 -> [w509]
              tunnel: w498 -> [w505]
              shift-right: [w513] -> w500
              shift-left: w501 -> [w508]
              tunnel: [w512] -> w497
              stop <- w515 continue-if-true
              n269 = call "Read Actual Position.vi"("error in (no error)"=w508, "Axis (1)"=w505, "VISA resource name"=w509) -> ("error out"=w506:errorcluster, "Position (units)"=w510:dbl, "VISA resource name out"=w507:refnum<visa-resource-name>)  [unwired: 2 in]
              n270 = local write "delay_pos"(w510) -> ()
              n271 = Decrement(x=w505) -> (x-1=w511:i32)
              n272 = call "Get Controller Status.vi"("error in (no error)"=w506, "VISA resource name"=w507) -> ("error out"=w513:errorcluster, "Controller Status"=w521:T5, "VISA resource name out"=w512:refnum<visa-resource-name>)  [unwired: 2 in, 1 out]
              n273 = Unbundle(w521) -> ("Axis1 moving"=w520:bool, "Axis2 moving"=w519:bool, "Axis3 moving"=w518:bool, "Axis4 moving"=w517:bool)  [unwired: 12 out]
              n274 = Build Array(w520, w519, w518, w517) -> (w516:bool[])
              n275 = Index Array(array=w516, index=w511) -> (element=w514:bool)
              n276 = Or(x=w514, y=w513) -> (x .or. y?=w515:bool)
            }
            n277 = Send Notification(notification=TRUE, notifier=w503, error in (no error)=w500) -> (error out=w504:errorcluster)  [unwired: 1 out]
          }
        }
      }
      frame "rel" {
        n278 = Dequeue Element(queue=w522) -> ()  [unwired: 2 in, 4 out]
        n279 = Fract/Exp String To Number(string=w530) -> (number=w524:dbl)  [unwired: 3 in, 1 out]
        n280 = call "Move Relative.vi"("error in (no error)"=w528, "Position (0 units)"=w524, "Axis (1)"=w525, "VISA resource name"=w529) -> ("error out"=w526:errorcluster, "VISA resource name out"=w527:refnum<visa-resource-name>)  [unwired: 2 in]
      }
      frame "release" {
        n281 = Dequeue Element(queue=w532) -> ()  [unwired: 2 in, 4 out]
        n282 = call "Close.vi"("error in (no error)"=w535, "VISA resource name"=w536) -> ("error out"=w533:errorcluster)  [unwired: 9 in]
      }
      frame "init" {
        n283 = Dequeue Element(queue=w542) -> ()  [unwired: 2 in, 4 out]
        n284 = call "Initialize.vi"("VISA resource name"="esp_visa", "Serial Link (RS232)"="Serial Link (RS232)") -> ("VISA resource name out"=w540:refnum<visa-resource-name>, "error out"=w541:errorcluster)  [unwired: 7 in]
      }
      frame "close" {
        n285 = Release Queue(queue=w544) -> ()  [unwired: 2 in, 3 out]
      }
    }
    "esp301" <- w452
    n286 = case shown="No Error" w452 {
      tunnel: [w466 -1] -> w458
      tunnel: w451 -> [w466 _]
      frame No Error {
      }
      frame Error {
      }
    }
  }
  n287 = while {
    tunnel: w22 -> [w556]
    shift-right: [w554] -> _
    shift-left: _ -> [w553]
    shift-right: [w551] -> _
    shift-left: -1 -> [w552]
    shift-right: [w550] -> _
    shift-left: _ -> [w549]
    tunnel: w21 -> [w548]
    stop <- w555 stop-if-true
    # "ISEG"
    n288 = Preview Queue Element(queue=w556, timeout in ms (-1)=w552) -> (element=w560:string)  [unwired: 1 in, 3 out]
    n289 = Match Pattern(string=w560, regular expression=":") -> (before substring=w558:string, after substring=w557:string)  [unwired: 1 in, 2 out]
    n290 = case shown="\"set\"" w558 {
      tunnel: w557 -> [_ w574 _ _ _]
      tunnel: w556 -> [_ w586 w628 w632 w636]
      tunnel: [_ _ _ _ TRUE] -> w555
      tunnel: [w563 w580 w626 w631 w633] -> w554
      tunnel: w553 -> [w565 w584 _ _ w633]
      tunnel: [0 _ _ _ _] -> w551
      tunnel: [w564 w581 T6 {"VISA Resource Name"="", "FP Notation"=FALSE, "Maximum Voltage"=0, "Maximum Current"=0} ("VISA Session Out") w629 w634] -> w550
      tunnel: w549 -> [w566 w585 w627 _ w634]
      tunnel: w548 -> [_ w569 _ _ _]
      frame "idle", Default {
        n291 = local read "Channel (A)"() -> (w567:enum16{"A", "B"})
        n292 = call "iseg NHQ xxx GetActualVoltage.vi"("error in (no error)"=w565, "Channel (A)"=w567, "VISA Session"=w566) -> ("error out"=w563:errorcluster, "Voltage"=w562:dbl, "VISA Session Out"=w564:T6)  [unwired: 5 in, 1 out]
        n293 = node(w562) -> (w561:dbl[unit])
        n294 = local write "Actual Voltage"(w561) -> ()
      }
      frame "set" {
        n295 = local read "Channel (A)"() -> (w577:enum16{"A", "B"})
        n296 = Dequeue Element(queue=w586) -> ()  [unwired: 2 in, 4 out]
        n297 = Match Pattern(string=w574, regular expression=":") -> (before substring=w573:string, after substring=w572:string)  [unwired: 1 in, 2 out]
        n298 = Fract/Exp String To Number(string=w573) -> (number=w576:dbl)  [unwired: 3 in, 1 out]
        n299 = call "iseg NHQ xxx SetNominalVoltage.vi"("error in (no error)"=w584, "Voltage (0 V)"=w576, "Channel (A)"=w577, "VISA Session"=w585) -> ("error out"=w587:errorcluster, "VISA Session Out"=w588:T6)  [unwired: 6 in]
        n300 = Equal?(x=w572, y="wait") -> (x = y?=w570:bool)
        n301 = call "iseg NHQ xxx StartVoltageChange.vi"("error in (no error)"=w587, "Channel (A)"=w577, "VISA Session"=w588) -> ("error out"=w582:errorcluster, "VISA Session Out"=w583:T6)  [unwired: 6 in, 1 out]
        n302 = case shown="True" w570 {
          tunnel: [w590 w600] -> w581
          tunnel: [w589 w592] -> w580
          tunnel: w583 -> [w590 w599]
          tunnel: w582 -> [w589 w598]
          tunnel: w576 -> [_ w597]
          tunnel: "volt_threshold" -> [_ w596]
          tunnel: "volt_timeout" -> [_ w595]
          tunnel: w577 -> [_ w594]
          tunnel: w569 -> [_ w593]
          frame False {
          }
          frame True {
            n303 = Tick Count (ms)() -> (millisecond timer value=w601:u32)
            n304 = while {
              shift-right: [w622] -> w600
              shift-left: w599 -> [w624]
              shift-right: [w609] -> w592
              shift-left: w598 -> [w623]
              tunnel: w594 -> [w621]
              tunnel: w596 -> [w618]
              tunnel: w601 -> [w616]
              tunnel: w595 -> [w614]
              tunnel: w597 -> [w613]
              tunnel: [w604] -> w591
              stop <- w610 stop-if-true
              n305 = Tick Count (ms)() -> (millisecond timer value=w617:u32)
              n306 = call "iseg NHQ xxx GetActualVoltage.vi"("error in (no error)"=w623, "Channel (A)"=w621, "VISA Session"=w624) -> ("error out"=w609:errorcluster, "Voltage"=w602:dbl, "VISA Session Out"=w622:T6)  [unwired: 5 in, 1 out]
              n307 = Absolute Value(x=w602) -> (abs(x)=w612:dbl)
              n308 = node(w602) -> (w603:dbl[unit])
              n309 = Subtract(x=w617, y=w616) -> (x-y=w615:u32)
              n310 = Subtract(x=w612, y=w613) -> (x-y=w620:dbl)
              n311 = local write "Actual Voltage"(w603) -> ()
              n312 = Absolute Value(x=w620) -> (abs(x)=w619:dbl)
              n313 = Greater?(x=w615, y=w614) -> (0:w608:bool)
              n314 = Less?(x=w619, y=w618) -> (x < y?=w611:bool)
              n315 = Or(x=w609, y=w608) -> (x .or. y?=w607:bool)
              n316 = Compound Arithmetic op=OR(w609, w611, w608) -> (w610:bool)
              n317 = Select(t="fail" ("element"), s=w607, f="done" ("element")) -> (s? t:f=w604:string)
            }
            n318 = Enqueue Element(queue=w593, element=w591) -> ()  [unwired: 2 in, 3 out]
          }
        }
      }
      frame "release" {
        n319 = Dequeue Element(queue=w628) -> ()  [unwired: 2 in, 4 out]
        n320 = call "iseg NHQ xxx Close.vi"("VISA session"=w627) -> ("error out"=w626:errorcluster)  [unwired: 14 in]
      }
      frame "init" {
        n321 = Dequeue Element(queue=w632) -> ()  [unwired: 2 in, 4 out]
        n322 = call "iseg NHQ xxx Initialize.vi"("VISA resource name"="VISA ISEG") -> ("VISA Session Out"=w629:T6, "error out"=w631:errorcluster)  [unwired: 13 in]
      }
      frame "close" {
        n323 = Release Queue(queue=w636) -> ()  [unwired: 2 in, 3 out]
      }
    }
    "error out" <- w554
  }
  n324 = while {
    tunnel: w21 -> [w644]
    tunnel: w28 -> [w643]
    tunnel: w27 -> [w641]
    tunnel: w22 -> [w640]
    tunnel: w18 -> [w639]
    tunnel: w15 -> [w638]
    tunnel: w1 -> [w637]
    stop <- w642 stop-if-true
    # "coherent"
    n325 = Preview Queue Element(queue=w644) -> (element=w648:string)  [unwired: 2 in, 3 out]
    n326 = Match Pattern(string=w648, regular expression=":") -> (before substring=w646:string, after substring=w645:string)  [unwired: 1 in, 2 out]
    n327 = case shown="\"volt\"" w646 {
      tunnel: w645 -> [_ _ _ _ _]
      tunnel: w644 -> [w650 w656 w681 w745 _]
      tunnel: w643 -> [w651 w652 w674 w743 _]
      tunnel: [TRUE _ _ _ _] -> w642
      tunnel: w641 -> [_ w655 w675 w742 _]
      tunnel: w640 -> [_ _ w676 _ _]
      tunnel: w639 -> [_ _ _ w759 _]
      tunnel: w638 -> [_ _ _ w740 _]
      tunnel: w637 -> [_ _ _ _ _]
      frame "close" {
        n328 = Release Queue(queue=w650) -> ()  [unwired: 2 in, 3 out]
        n329 = Release Queue(queue=w651) -> ()  [unwired: 2 in, 3 out]
      }
      frame "single" {
        n330 = Dequeue Element(queue=w656) -> (error out=w653:errorcluster)  [unwired: 2 in, 3 out]
        n331 = Flush Queue(queue=w652, error in (no error)=w653) -> (error out=w654:errorcluster)  [unwired: 2 out]
        n332 = while {
          tunnel: w655 -> [w660]
          tunnel: w654 -> [w659]
          tunnel: w652 -> [w658]
          stop <- w657 continue-if-true
          n333 = flat-sequence {
            tunnel: w660 -> [w665]
            tunnel: w659 -> [w662]
            tunnel: w658 -> [w661]
            tunnel: ["continous acq."] -> w657
            frame #0 {
              n334 = Enqueue Element(queue=w665, element="snap", error in (no error)=w662) -> (error out=w663:errorcluster)  [unwired: 1 in, 2 out]
              n335 = Dequeue Element(queue=w661, error in (no error)=w663) -> ()  [unwired: 1 in, 4 out]
            }
            frame #1 {
            }
          }
        }
      }
      frame "volt" {
        n336 = Flush Queue(queue=w681) -> (queue out=w677:refnum<queue>)  [unwired: 1 in, 2 out]
        n337 = local read "Path"() -> (w680:path)
        n338 = Build Path(base path=w680, name or relative path="head") -> (appended path=w669:path)
        n339 = Build Path(base path=w669, name or relative path="raw") -> (appended path=w671:path)
        n340 = Build Path(base path=w669, name or relative path="LUT.txt") -> (appended path=w672:path)
        n341 = Create Folder(path (use dialog)=w671) -> (created path=w670:path)  [unwired: 2 in, 2 out]
        n342 = for {
          N: "iterations 2" -> [_]
          tunnel: w677 -> [w683]
          tunnel: w676 -> [w694]
          tunnel: w675 -> [w693]
          tunnel: w674 -> [w692]
          tunnel: w672 -> [w687]
          tunnel: w670 -> [w686]
          shift-right: [w682] -> _
          shift-left: _ -> [w685]
          tunnel: [w683] -> w668
          i -> [w691]
          n343 = call-poly <vilib>:"Ramp Pattern.vi"("start"="volt_start", "end"="volt_end", "samples"="volt_samples") -> ("Ramp Pattern"=w690:dbl[])  [unwired: 7 in, 1 out]
          n344 = Array Size(array=w690) -> (size(s)=w689:i32)
          n345 = Number To Fractional String(number=w690) -> (F-format string=w696:string[])  [unwired: 3 in]
          n346 = Multiply(x=w689, y=w691) -> (x*y=w688:i32)
          n347 = for {
            N -> [w704]
            tunnel: w683 -> [_]
            tunnel: w696 -> [w715] mode=indexing
            tunnel: "set:" ("element") -> [w726]
            tunnel: w694 -> [w725]
            tunnel: w683 -> [w723]
            tunnel: w693 -> [w721]
            tunnel: w692 -> [w719]
            shift-right: [w706] -> w682
            shift-left: w685 -> [w718]
            tunnel: w688 -> [w717]
            tunnel: w687 -> [w714]
            tunnel: w686 -> [w713]
            tunnel: ":wait" ("element") -> [w705]
            i -> [w703]
            n348 = Concatenate Strings(w726, w715, w705) -> (w727:string)
            n349 = Add(x=w717, y=w703) -> (x+y=w716:i32)
            n350 = Divide(x=w703, y=w704) -> (x/y=→"Slide 2":dbl)
            n351 = Number To Decimal String(number=w716) -> (decimal integer string=w712:string)  [unwired: 1 in]
            n352 = Enqueue Element(queue=w725, element=w727, error in (no error)=w718) -> (error out=w724:errorcluster)  [unwired: 1 in, 2 out]
            n353 = Dequeue Element(queue=w723, error in (no error)=w724) -> (element=w709:string, error out=w708:errorcluster)  [unwired: 1 in, 2 out]
            n354 = Equal?(x="stop" ("y"), y=w709) -> (x = y?=w707:bool)
            n355 = call "inject_error.vi"("error in"=w708, "s"=w707) -> ("error out"=w700:errorcluster)  [unwired: 9 in]
            n356 = Enqueue Element(queue=w721, element="snap", error in (no error)=w700) -> (error out=w720:errorcluster)  [unwired: 1 in, 2 out]
            n357 = Dequeue Element(queue=w719, error in (no error)=w720) -> (element=w711:dbl[][], error out=w701:errorcluster)  [unwired: 1 in, 2 out]
            n358 = case shown="No Error" w701 {
              selector: w701 -> [w730 w737]
              tunnel: w715 -> [w728 _]
              tunnel: w714 -> [w735 _]
              tunnel: w713 -> [w734 _]
              tunnel: w712 -> [w733 _]
              tunnel: w711 -> [w731 _]
              tunnel: [w730 w737] -> w706
              frame No Error {
                n359 = Build Path(base path=w734, name or relative path=w733) -> (appended path=w732:path)
                n360 = Write to Binary File(file (use dialog)=w732, data=w731) -> ()  [unwired: 4 in, 3 out]
                n361 = Build Array(w733, w728) -> (w729:string[])
                n362 = call-poly <vilib>:"Write Delimited Spreadsheet.vi"("file path (dialog if empty)"=w735, "1D data"=w729, "append to file? (new file:F)"=TRUE) -> ()  [unwired: 11 in, 2 out]
              }
              frame Error {
              }
            }
          }
        }
        n363 = Flush Queue(queue=w668) -> ()  [unwired: 1 in, 3 out]
      }
      frame "delay" {
        n364 = local read "Path"() -> (w758:path)
        n365 = Dequeue Element(queue=w745) -> ()  [unwired: 2 in, 4 out]
        n366 = Build Path(base path=w758, name or relative path="delayscan_header") -> (appended path=w747:path)
        n367 = call <vilib>:"Check if File or Folder Exists.vi"("path"=w747) -> ("file or folder exists?"=w749:bool, "dup path"=w748:path)  [unwired: 8 in, 1 out]
        n368 = case shown="False" w749 {
          tunnel: [w891 w892] -> w746
          tunnel: w748 -> [w890 w892]
          frame False {
            n369 = Create Folder(path (use dialog)=w890) -> (created path=w891:path)  [unwired: 2 in, 2 out]
          }
          frame True {
          }
        }
        n370 = call "create scan vectr.vi"("Table Control"="waypoints") -> ("Array"=w750:dbl[])
        n371 = Flush Queue(queue=w743) -> (queue out=w744:refnum<queue>)  [unwired: 1 in, 2 out]
        n372 = Array Size(array=w750) -> (size(s)=w753:i32)
        n373 = Build Path(base path=w746, name or relative path="times.txt") -> (appended path=w755:path)
        n374 = Flush Queue(queue=w740) -> (queue out=w739:refnum<queue>)  [unwired: 1 in, 2 out]
        n375 = Flush Queue(queue=w742) -> (queue out=w741:refnum<queue>)  [unwired: 1 in, 2 out]
        n376 = Get Date/Time In Seconds() -> (seconds since 1Jan1904=w738:timestamp)
        n377 = Initialize Array(0.0 ("element"), w753) -> (w751:dbl[])
        n378 = call-poly <vilib>:"Write Delimited Spreadsheet.vi"("file path (dialog if empty)"=w755, "1D data"=w750, "transpose? (no:F)"=TRUE) -> ()  [unwired: 11 in, 2 out]
        n379 = while {
          tunnel: w750 -> [w772]
          tunnel: w739 -> [w776]
          tunnel: w759 -> [w775]
          tunnel: w744 -> [w774]
          tunnel: w741 -> [w773]
          tunnel: w746 -> [w771]
          shift-right: [w769] -> _
          shift-left: w751 -> [w770]
          tunnel: w746 -> [w768]
          tunnel: w738 -> [w762]
          i -> [w766]
          stop <- w763 stop-if-true
          n380 = for {
            N -> [w787]
            tunnel: w772 -> [w793] mode=indexing
            tunnel: w776 -> [w857]
            tunnel: w775 -> [w855]
            tunnel: w774 -> [w853]
            tunnel: w773 -> [w851]
            tunnel: w772 -> [w821]
            tunnel: w771 -> [w849]
            tunnel: w766 -> [w791]
            shift-right: [w819] -> w769
            shift-left: w770 -> [w822]
            tunnel: w768 -> [w817]
            tunnel: [w792] -> w765
            tunnel: w762 -> [w785]
            tunnel: "iterations" -> [w788]
            i -> [w783]
            stop <- w792 stop-if-true
            n381 = Multiply(x=w787, y=w791) -> (x*y=w790:i32)
            n382 = local read "t0 @"() -> (w862:dbl)
            n383 = Get Date/Time In Seconds() -> (seconds since 1Jan1904=w789:timestamp)
            n384 = Get Date/Time In Seconds() -> (seconds since 1Jan1904=w798:timestamp)
            n385 = Add(x=w790, y=w783) -> (x+y=w777:i32)
            n386 = Divide(x=w791, y=10000) -> (x/y=w847:dbl)
            n387 = Subtract(x=w785, y=w789) -> (x-y=w786:dbl)
            n388 = Format Date/Time String(time format string (%c)="DelayScan_%Y%m%d_%H%M%S_", seconds (now)=w798) -> (date/time string=w794:string)  [unwired: 1 in]
            n389 = Divide(x=w786, y=w777) -> (x/y=w781:dbl)
            n390 = Multiply(x=w788, y=w787) -> (x*y=w784:i32)
            n391 = Divide(x=w783, y=10000) -> (x/y=w804:dbl)
            n392 = Number To Fractional String(number=w847) -> (F-format string=w846:string)  [unwired: 3 in]
            n393 = call "time2mm.vi"("fs[1]/ps[0]"=TRUE, "Offset (mm)"=w862, "time"=w793) -> ("position (mm)"=w801:dbl)
            n394 = Number To Fractional String(number=w804) -> (F-format string=w842:string)  [unwired: 3 in]
            n395 = Subtract(x=w784, y=w777) -> (x-y=w782:i32)
            n396 = local write "delayscan_time/step"(w781) -> ()
            n397 = Multiply(x=w781, y=w782) -> (x*y=w780:dbl)
            n398 = Number To Fractional String(number=w801) -> (F-format string=w860:string)  [unwired: 3 in]
            n399 = String Subset(string=w846, offset (0)=2, length (rest)=4 ("length (rest)")) -> (substring=w844:string)
            n400 = local write "duration"(w780) -> ()
            n401 = String Subset(string=w842, offset (0)=2, length (rest)=4 ("length (rest)")) -> (substring=w796:string)
            n402 = Concatenate Strings("abs:" ("string"), w860, ":confirm" ("string")) -> (w858:string)
            n403 = Build Path(base path=w849, name or relative path=w844) -> (appended path=w807:path)
            n404 = call <vilib>:"Check if File or Folder Exists.vi"("path"=w807) -> ("file or folder exists?"=w808:bool, "dup path"=w809:path)  [unwired: 8 in, 1 out]
            n405 = Concatenate Strings(w794, w796) -> (w797:string)
            n406 = case shown="False" w808 {
              tunnel: [w888 w889] -> w806
              tunnel: w809 -> [w887 w889]
              frame False {
                n407 = Create Folder(path (use dialog)=w887) -> (created path=w888:path)  [unwired: 2 in, 2 out]
              }
              frame True {
              }
            }
            n408 = Enqueue Element(queue=w857, element=w858) -> (error out=w856:errorcluster)  [unwired: 2 in, 2 out]
            n409 = Concatenate Strings(w797, ".bin" ("string")) -> (w813:string)
            n410 = Concatenate Strings(w797, ".png" ("string")) -> (w811:string)
            n411 = Wait on Notification(notifier=w855, error in (no error)=w856) -> (error out=w854:errorcluster)  [unwired: 2 in, 3 out]
            n412 = Build Path(base path=w806, name or relative path=w813) -> (appended path=w818:path)
            n413 = Build Path(base path=w817, name or relative path="positions.txt") -> (appended path=w815:path)
            n414 = property on="live" class="IntGraph (strict)"() -> ("CrsrLis"=w841:T7)  [unwired: 2 in, 2 out]
            n415 = Build Path(base path=w806, name or relative path=w811) -> (appended path=w810:path)
            n416 = Enqueue Element(queue=w851, element="snap", error in (no error)=w854) -> (error out=w852:errorcluster)  [unwired: 1 in, 2 out]
            n417 = Index Array(array=w841) -> (element #1=w840:T8, element #2=w839:T8)  [unwired: 2 in]
            n418 = Unbundle By Name(w840) -> ("Position.X"=w838:dbl, "Position.Y"=w836:dbl)
            n419 = Unbundle By Name(w839) -> ("Position.X"=w837:dbl, "Position.Y"=w835:dbl)
            n420 = Dequeue Element(queue=w853, error in (no error)=w852) -> (element=w779:dbl[][])  [unwired: 1 in, 3 out]
            n421 = Build Array(w838, w837) -> (w834:dbl[])
            n422 = Build Array(w836, w835) -> (w833:dbl[])
            n423 = Array Max & Min(array=w834) -> (max value=w832:dbl, min value=w830:dbl)  [unwired: 2 out]
            n424 = Array Max & Min(array=w833) -> (max value=w831:dbl, min value=w828:dbl)  [unwired: 2 out]
            n425 = while {
              tunnel: ["delayscan_stop"] -> w792
              tunnel: w779 -> [w864]
              tunnel: [w864] -> w778
              stop <- "delayscan_pause" continue-if-true
              n426 = Wait (ms)(milliseconds to wait=u32 100) -> ()  [unwired: 1 out]
            }
            n427 = Write to Binary File(file (use dialog)=w818, data=w778) -> ()  [unwired: 4 in, 3 out]
            n428 = Subtract(x=w830, y=w832) -> (x-y=w829:dbl)
            n429 = Subtract(x=w828, y=w831) -> (x-y=w827:dbl)
            n430 = Array Subset(array=w778, index (row)=w830, length (row)=w829, index (col)=w828, length (col)=w827) -> (w826:dbl[][])
            n431 = Array Size(array=w778) -> (size(s)=w824:i32[])
            n432 = Add Array Elements(numeric array=w826) -> (sum=w825:dbl)
            n433 = Multiply Array Elements(1:w824) -> (0:w823:i32)
            n434 = Divide(x=w825, y=w823) -> ()  [unwired: 1 out]
            n435 = disable-structure shown="Disabled" {
              disable-tunnel: w810 -> [w869 _]
              disable-tunnel: w778 -> [w868 _]
              frame Disabled {
                w883 = T2 7 items=["Grayscale (U8)", "Grayscale (I16)", "Grayscale (SGL)", "Complex (CSG)", "RGB (U32)", "HSL (U32)", "RGB (U64)", "Grayscale (U16)"] ("Image Type")
                n436 = for {
                  tunnel: w868 -> [w886] mode=indexing
                  tunnel: [w885] -> w878 mode=indexing
                  n437 = Reverse 1D Array(array=w886) -> (reversed array=w885:dbl[])
                }
                n438 = Transpose 2D Array(2D array=w878) -> (transposed array=w872:dbl[][])
                n439 = Array Max & Min(array=w872) -> (min value=w871:dbl)  [unwired: 3 out]
                n440 = Subtract(x=w872, y=w871) -> (x-y=w870:dbl[][])
                n441 = call "IMAQ Create"("Image Name"="untitled", "Image Type"=w883) -> ("New Image"=w884:T3)  [unwired: 3 in, 1 out]
                n442 = Array Max & Min(array=w870) -> (max value=w877:dbl)  [unwired: 3 out]
                n443 = Divide(x=w870, y=w877) -> (x/y=w876:dbl[][])
                n444 = Multiply(x=w876, y=255) -> (x*y=w874:dbl[][])
                n445 = To Unsigned Word Integer(number=w874) -> (unsigned 16bit integer=w873:u16[][])
                n446 = call "IMAQ ArrayToImage"("Image Pixels (U16)"=w873, "Image"=w884) -> ("Image Out"=w882:T3)  [unwired: 8 in, 1 out]
                n447 = call-poly "IMAQ Write File 2"("Image Quality"=u32 1000, "File Path"=w869, "Image"=w882) -> ("Image Out (duplicate)"=w880:T3)  [unwired: 7 in, 1 out]
                n448 = call "IMAQ Dispose"("Image"=w880) -> ()  [unwired: 5 in, 1 out]
              }
              frame Enabled {
              }
            }
            n449 = Replace Array Subset(array=w822, new element=w801, index=w783) -> (w819:dbl[])
            n450 = Bundle("Array"=w821, w819) -> (→"XY Graph":cluster{"Array":dbl[], dbl[]})  [unwired: 1 in]
            n451 = call-poly <vilib>:"Write Delimited Spreadsheet.vi"("file path (dialog if empty)"=w815, "format (%.3f)"="%.6f", "1D data"=w819, "transpose? (no:F)"=TRUE) -> ()  [unwired: 10 in, 2 out]
          }
          n452 = Increment(x=w766) -> (x+1=w767:i32)
          n453 = Greater Or Equal?(x=w767, y="iterations") -> (x >= y?=w764:bool)
          n454 = Or(x=w765, y=w764) -> (x .or. y?=w763:bool)
        }
      }
      frame "idle", Default {
      }
    }
  }
